vi "BackgroundCorrect.vi"(0 "Load Images":path=path "F:/pHGradienten/2015/150416_Bindungskurve_FeCN/500uW/15/a000000.tif", 1 "Load Background Images":path=path "F:/pHGradienten/2015/150218_ssDNA/ATTO488/50mer_2/a000000.tif", 2 "Image":dbl[][](graph), 3 "Frame":i32, 4 "Binning":dbl, 5 "Background Correction Mode:":T1(ring)=enum."Constant Value", 6 "# of Background image":i32=1499, 8 "Offset":dbl, 9 "Constant":dbl) -> (7 "Corrected Image":dbl[][](graph))   [LabVIEW 2010]
panel:
  out "Background Path in Folder":path[](array[path])=[path "F:/pHGradienten/2015/150416_Bindungskurve_FeCN/500uW/10/a000001.tif", path "F:/pHGradienten/2015/150416_Bindungskurve_FeCN/500uW/10/a000002.tif", path "F:/pHGradienten/2015/150416_Bindungskurve_FeCN/500uW/10/a000003.tif", path "F:/pHGradienten/2015/150416_Bindungskurve_FeCN/500uW/10/a000004.tif", path "F:/pHGradienten/2015/150416_Bindungskurve_FeCN/500uW/10/a000005.tif", path "F:/pHGradienten/2015/150416_Bindungskurve_FeCN/500uW/10/a000006.tif", path "F:/pHGradienten/2015/150416_Bindungskurve_FeCN/500uW/10/a000007.tif", path "F:/pHGradienten/2015/150416_Bindungskurve_FeCN/500uW/10/a000008.tif", path "F:/pHGradienten/2015/150416_Bindungskurve_FeCN/500uW/10/a000009.tif", path "F:/pHGradienten/2015/150416_Bindungskurve_FeCN/500uW/10/a000010.tif", path "F:/pHGradienten/2015/150416_Bindungskurve_FeCN/500uW/10/a000011.tif", path "F:/pHGradienten/2015/150416_Bindungskurve_FeCN/500uW/10/a000012.tif", path "F:/pHGradienten/2015/150416_Bindungskurve_FeCN/500uW/10/a000013.tif", path "F:/pHGradienten/2015/150416_Bindungskurve_FeCN/500uW/10/a000014.tif", path "F:/pHGradienten/2015/150416_Bindungskurve_FeCN/500uW/10/a000015.tif", path "F:/pHGradienten/2015/150416_Bindungskurve_FeCN/500uW/10/a000016.tif", path "F:/pHGradienten/2015/150416_Bindungskurve_FeCN/500uW/10/a000017.tif", path "F:/pHGradienten/2015/150416_Bindungskurve_FeCN/500uW/10/a000018.tif", path "F:/pHGradienten/2015/150416_Bindungskurve_FeCN/500uW/10/a000019.tif", path "F:/pHGradienten/2015/150416_Bindungskurve_FeCN/500uW/10/a000020.tif", path "F:/pHGradienten/2015/150416_Bindungskurve_FeCN/500uW/10/a000021.tif", path "F:/pHGradienten/2015/150416_Bindungskurve_FeCN/500uW/10/a000022.tif", path "F:/pHGradienten/2015/150416_Bindungskurve_FeCN/500uW/10/a000023.tif", path "F:/pHGradienten/2015/150416_Bindungskurve_FeCN/500uW/10/a000024.tif", path "F:/pHGradienten/2015/150416_Bindungskurve_FeCN/500uW/10/a000025.tif", path "F:/pHGradienten/2015/150416_Bindungskurve_FeCN/500uW/10/a000026.tif", path "F:/pHGradienten/2015/150416_Bindungskurve_FeCN/500uW/10/a000027.tif", path "F:/pHGradienten/2015/150416_Bindungskurve_FeCN/500uW/10/a000028.tif", path "F:/pHGradienten/2015/150416_Bindungskurve_FeCN/500uW/10/a000029.tif", path "F:/pHGradienten/2015/150416_Bindungskurve_FeCN/500uW/10/a000030.tif", path "F:/pHGradienten/2015/150416_Bindungskurve_FeCN/500uW/10/a000031.tif", path "F:/pHGradienten/2015/150416_Bindungskurve_FeCN/500uW/10/a000032.tif", path "F:/pHGradienten/2015/150416_Bindungskurve_FeCN/500uW/10/a000033.tif", path "F:/pHGradienten/2015/150416_Bindungskurve_FeCN/500uW/10/a000034.tif", path "F:/pHGradienten/2015/150416_Bindungskurve_FeCN/500uW/10/a000035.tif", path "F:/pHGradienten/2015/150416_Bindungskurve_FeCN/500uW/10/a000036.tif", path "F:/pHGradienten/2015/150416_Bindungskurve_FeCN/500uW/10/a000037.tif", path "F:/pHGradienten/2015/150416_Bindungskurve_FeCN/500uW/10/a000038.tif", path "F:/pHGradienten/2015/150416_Bindungskurve_FeCN/500uW/10/a000039.tif", path "F:/pHGradienten/2015/150416_Bindungskurve_FeCN/500uW/10/a000040.tif", path "F:/pHGradienten/2015/150416_Bindungskurve_FeCN/500uW/10/a000041.tif", path "F:/pHGradienten/2015/150416_Bindungskurve_FeCN/500uW/10/a000042.tif", path "F:/pHGradienten/2015/150416_Bindungskurve_FeCN/500uW/10/a000043.tif", path "F:/pHGradienten/2015/150416_Bindungskurve_FeCN/500uW/10/a000044.tif", path "F:/pHGradienten/2015/150416_Bindungskurve_FeCN/500uW/10/a000045.tif", path "F:/pHGradienten/2015/150416_Bindungskurve_FeCN/500uW/10/a000046.tif", path "F:/pHGradienten/2015/150416_Bindungskurve_FeCN/500uW/10/a000047.tif", path "F:/pHGradienten/2015/150416_Bindungskurve_FeCN/500uW/10/a000048.tif", path "F:/pHGradienten/2015/150416_Bindungskurve_FeCN/500uW/10/a000049.tif", path "F:/pHGradienten/2015/150416_Bindungskurve_FeCN/500uW/10/a000050.tif", path "F:/pHGradienten/2015/150416_Bindungskurve_FeCN/500uW/10/a000051.tif", path "F:/pHGradienten/2015/150416_Bindungskurve_FeCN/500uW/10/a000052.tif", path "F:/pHGradienten/2015/150416_Bindungskurve_FeCN/500uW/10/a000053.tif", path "F:/pHGradienten/2015/150416_Bindungskurve_FeCN/500uW/10/a000054.tif", path "F:/pHGradienten/2015/150416_Bindungskurve_FeCN/500uW/10/a000055.tif", path "F:/pHGradienten/2015/150416_Bindungskurve_FeCN/500uW/10/a000056.tif", path "F:/pHGradienten/2015/150416_Bindungskurve_FeCN/500uW/10/a000057.tif", path "F:/pHGradienten/2015/150416_Bindungskurve_FeCN/500uW/10/a000058.tif", path "F:/pHGradienten/2015/150416_Bindungskurve_FeCN/500uW/10/a000059.tif", path "F:/pHGradienten/2015/150416_Bindungskurve_FeCN/500uW/10/a000060.tif", path "F:/pHGradienten/2015/150416_Bindungskurve_FeCN/500uW/10/a000061.tif", path "F:/pHGradienten/2015/150416_Bindungskurve_FeCN/500uW/10/a000062.tif", path "F:/pHGradienten/2015/150416_Bindungskurve_FeCN/500uW/10/a000063.tif", path "F:/pHGradienten/2015/150416_Bindungskurve_FeCN/500uW/10/a000064.tif", path "F:/pHGradienten/2015/150416_Bindungskurve_FeCN/500uW/10/a000065.tif", path "F:/pHGradienten/2015/150416_Bindungskurve_FeCN/500uW/10/a000066.tif", path "F:/pHGradienten/2015/150416_Bindungskurve_FeCN/500uW/10/a000067.tif", path "F:/pHGradienten/2015/150416_Bindungskurve_FeCN/500uW/10/a000068.tif", path "F:/pHGradienten/2015/150416_Bindungskurve_FeCN/500uW/10/a000069.tif", path "F:/pHGradienten/2015/150416_Bindungskurve_FeCN/500uW/10/a000070.tif", path "F:/pHGradienten/2015/150416_Bindungskurve_FeCN/500uW/10/a000071.tif", path "F:/pHGradienten/2015/150416_Bindungskurve_FeCN/500uW/10/a000072.tif", path "F:/pHGradienten/2015/150416_Bindungskurve_FeCN/500uW/10/a000073.tif", path "F:/pHGradienten/2015/150416_Bindungskurve_FeCN/500uW/10/a000074.tif", path "F:/pHGradienten/2015/150416_Bindungskurve_FeCN/500uW/10/a000075.tif", path "F:/pHGradienten/2015/150416_Bindungskurve_FeCN/500uW/10/a000076.tif", path "F:/pHGradienten/2015/150416_Bindungskurve_FeCN/500uW/10/a000077.tif", path "F:/pHGradienten/2015/150416_Bindungskurve_FeCN/500uW/10/a000078.tif", path "F:/pHGradienten/2015/150416_Bindungskurve_FeCN/500uW/10/a000079.tif", path "F:/pHGradienten/2015/150416_Bindungskurve_FeCN/500uW/10/a000080.tif", path "F:/pHGradienten/2015/150416_Bindungskurve_FeCN/500uW/10/a000081.tif", path "F:/pHGradienten/2015/150416_Bindungskurve_FeCN/500uW/10/a000082.tif", path "F:/pHGradienten/2015/150416_Bindungskurve_FeCN/500uW/10/a000083.tif", path "F:/pHGradienten/2015/150416_Bindungskurve_FeCN/500uW/10/a000084.tif", path "F:/pHGradienten/2015/150416_Bindungskurve_FeCN/500uW/10/a000085.tif", path "F:/pHGradienten/2015/150416_Bindungskurve_FeCN/500uW/10/a000086.tif", path "F:/pHGradienten/2015/150416_Bindungskurve_FeCN/500uW/10/a000087.tif", path "F:/pHGradienten/2015/150416_Bindungskurve_FeCN/500uW/10/a000088.tif", path "F:/pHGradienten/2015/150416_Bindungskurve_FeCN/500uW/10/a000089.tif", path "F:/pHGradienten/2015/150416_Bindungskurve_FeCN/500uW/10/a000090.tif", path "F:/pHGradienten/2015/150416_Bindungskurve_FeCN/500uW/10/a000091.tif", path "F:/pHGradienten/2015/150416_Bindungskurve_FeCN/500uW/10/a000092.tif", path "F:/pHGradienten/2015/150416_Bindungskurve_FeCN/500uW/10/a000093.tif", path "F:/pHGradienten/2015/150416_Bindungskurve_FeCN/500uW/10/a000094.tif", path "F:/pHGradienten/2015/150416_Bindungskurve_FeCN/500uW/10/a000095.tif", path "F:/pHGradienten/2015/150416_Bindungskurve_FeCN/500uW/10/a000096.tif", path "F:/pHGradienten/2015/150416_Bindungskurve_FeCN/500uW/10/a000097.tif", path "F:/pHGradienten/2015/150416_Bindungskurve_FeCN/500uW/10/a000098.tif", path "F:/pHGradienten/2015/150416_Bindungskurve_FeCN/500uW/10/a000099.tif", path "F:/pHGradienten/2015/150416_Bindungskurve_FeCN/500uW/10/a000100.tif", path "F:/pHGradienten/2015/150416_Bindungskurve_FeCN/500uW/10/a000101.tif", path "F:/pHGradienten/2015/150416_Bindungskurve_FeCN/500uW/10/a000102.tif", path "F:/pHGradienten/2015/150416_Bindungskurve_FeCN/500uW/10/a000103.tif", path "F:/pHGradienten/2015/150416_Bindungskurve_FeCN/500uW/10/a000104.tif", path "F:/pHGradienten/2015/150416_Bindungskurve_FeCN/500uW/10/a000105.tif", path "F:/pHGradienten/2015/150416_Bindungskurve_FeCN/500uW/10/a000106.tif", path "F:/pHGradienten/2015/150416_Bindungskurve_FeCN/500uW/10/a000107.tif", path "F:/pHGradienten/2015/150416_Bindungskurve_FeCN/500uW/10/a000108.tif", path "F:/pHGradienten/2015/150416_Bindungskurve_FeCN/500uW/10/a000109.tif", path "F:/pHGradienten/2015/150416_Bindungskurve_FeCN/500uW/10/a000110.tif", path "F:/pHGradienten/2015/150416_Bindungskurve_FeCN/500uW/10/a000111.tif", path "F:/pHGradienten/2015/150416_Bindungskurve_FeCN/500uW/10/a000112.tif", path "F:/pHGradienten/2015/150416_Bindungskurve_FeCN/500uW/10/a000113.tif", path "F:/pHGradienten/2015/150416_Bindungskurve_FeCN/500uW/10/a000114.tif", path "F:/pHGradienten/2015/150416_Bindungskurve_FeCN/500uW/10/a000115.tif", path "F:/pHGradienten/2015/150416_Bindungskurve_FeCN/500uW/10/a000116.tif", path "F:/pHGradienten/2015/150416_Bindungskurve_FeCN/500uW/10/a000117.tif", path "F:/pHGradienten/2015/150416_Bindungskurve_FeCN/500uW/10/a000118.tif", path "F:/pHGradienten/2015/150416_Bindungskurve_FeCN/500uW/10/a000119.tif", path "F:/pHGradienten/2015/150416_Bindungskurve_FeCN/500uW/10/a000120.tif", path "F:/pHGradienten/2015/150416_Bindungskurve_FeCN/500uW/10/a000121.tif", path "F:/pHGradienten/2015/150416_Bindungskurve_FeCN/500uW/10/a000122.tif", path "F:/pHGradienten/2015/150416_Bindungskurve_FeCN/500uW/10/a000123.tif", path "F:/pHGradienten/2015/150416_Bindungskurve_FeCN/500uW/10/a000124.tif", path "F:/pHGradienten/2015/150416_Bindungskurve_FeCN/500uW/10/a000125.tif", path "F:/pHGradienten/2015/150416_Bindungskurve_FeCN/500uW/10/a000126.tif", path "F:/pHGradienten/2015/150416_Bindungskurve_FeCN/500uW/10/a000127.tif", path "F:/pHGradienten/2015/150416_Bindungskurve_FeCN/500uW/10/a000128.tif", path "F:/pHGradienten/2015/150416_Bindungskurve_FeCN/500uW/10/a000129.tif", path "F:/pHGradienten/2015/150416_Bindungskurve_FeCN/500uW/10/a000130.tif", path "F:/pHGradienten/2015/150416_Bindungskurve_FeCN/500uW/10/a000131.tif", path "F:/pHGradienten/2015/150416_Bindungskurve_FeCN/500uW/10/a000132.tif", path "F:/pHGradienten/2015/150416_Bindungskurve_FeCN/500uW/10/a000133.tif", path "F:/pHGradienten/2015/150416_Bindungskurve_FeCN/500uW/10/a000134.tif", path "F:/pHGradienten/2015/150416_Bindungskurve_FeCN/500uW/10/a000135.tif", path "F:/pHGradienten/2015/150416_Bindungskurve_FeCN/500uW/10/a000136.tif", path "F:/pHGradienten/2015/150416_Bindungskurve_FeCN/500uW/10/a000137.tif", path "F:/pHGradienten/2015/150416_Bindungskurve_FeCN/500uW/10/a000138.tif", path "F:/pHGradienten/2015/150416_Bindungskurve_FeCN/500uW/10/a000139.tif", path "F:/pHGradienten/2015/150416_Bindungskurve_FeCN/500uW/10/a000140.tif", path "F:/pHGradienten/2015/150416_Bindungskurve_FeCN/500uW/10/a000141.tif", path "F:/pHGradienten/2015/150416_Bindungskurve_FeCN/500uW/10/a000142.tif", path "F:/pHGradienten/2015/150416_Bindungskurve_FeCN/500uW/10/a000143.tif", path "F:/pHGradienten/2015/150416_Bindungskurve_FeCN/500uW/10/a000144.tif", path "F:/pHGradienten/2015/150416_Bindungskurve_FeCN/500uW/10/a000145.tif", path "F:/pHGradienten/2015/150416_Bindungskurve_FeCN/500uW/10/a000146.tif", path "F:/pHGradienten/2015/150416_Bindungskurve_FeCN/500uW/10/a000147.tif", path "F:/pHGradienten/2015/150416_Bindungskurve_FeCN/500uW/10/a000148.tif", path "F:/pHGradienten/2015/150416_Bindungskurve_FeCN/500uW/10/a000149.tif", path "F:/pHGradienten/2015/150416_Bindungskurve_FeCN/500uW/10/a000150.tif", path "F:/pHGradienten/2015/150416_Bindungskurve_FeCN/500uW/10/a000151.tif", path "F:/pHGradienten/2015/150416_Bindungskurve_FeCN/500uW/10/a000152.tif", path "F:/pHGradienten/2015/150416_Bindungskurve_FeCN/500uW/10/a000153.tif", path "F:/pHGradienten/2015/150416_Bindungskurve_FeCN/500uW/10/a000154.tif", path "F:/pHGradienten/2015/150416_Bindungskurve_FeCN/500uW/10/a000155.tif", path "F:/pHGradienten/2015/150416_Bindungskurve_FeCN/500uW/10/a000156.tif", path "F:/pHGradienten/2015/150416_Bindungskurve_FeCN/500uW/10/a000157.tif", path "F:/pHGradienten/2015/150416_Bindungskurve_FeCN/500uW/10/a000158.tif", path "F:/pHGradienten/2015/150416_Bindungskurve_FeCN/500uW/10/a000159.tif", path "F:/pHGradienten/2015/150416_Bindungskurve_FeCN/500uW/10/a000160.tif", path "F:/pHGradienten/2015/150416_Bindungskurve_FeCN/500uW/10/a000161.tif", path "F:/pHGradienten/2015/150416_Bindungskurve_FeCN/500uW/10/a000162.tif", path "F:/pHGradienten/2015/150416_Bindungskurve_FeCN/500uW/10/a000163.tif", path "F:/pHGradienten/2015/150416_Bindungskurve_FeCN/500uW/10/a000164.tif", path "F:/pHGradienten/2015/150416_Bindungskurve_FeCN/500uW/10/a000165.tif", path "F:/pHGradienten/2015/150416_Bindungskurve_FeCN/500uW/10/a000166.tif", path "F:/pHGradienten/2015/150416_Bindungskurve_FeCN/500uW/10/a000167.tif", path "F:/pHGradienten/2015/150416_Bindungskurve_FeCN/500uW/10/a000168.tif", path "F:/pHGradienten/2015/150416_Bindungskurve_FeCN/500uW/10/a000169.tif", path "F:/pHGradienten/2015/150416_Bindungskurve_FeCN/500uW/10/a000170.tif", path "F:/pHGradienten/2015/150416_Bindungskurve_FeCN/500uW/10/a000171.tif", path "F:/pHGradienten/2015/150416_Bindungskurve_FeCN/500uW/10/a000172.tif", path "F:/pHGradienten/2015/150416_Bindungskurve_FeCN/500uW/10/a000173.tif", path "F:/pHGradienten/2015/150416_Bindungskurve_FeCN/500uW/10/a000174.tif", path "F:/pHGradienten/2015/150416_Bindungskurve_FeCN/500uW/10/a000175.tif", path "F:/pHGradienten/2015/150416_Bindungskurve_FeCN/500uW/10/a000176.tif", path "F:/pHGradienten/2015/150416_Bindungskurve_FeCN/500uW/10/a000177.tif", path "F:/pHGradienten/2015/150416_Bindungskurve_FeCN/500uW/10/a000178.tif", path "F:/pHGradienten/2015/150416_Bindungskurve_FeCN/500uW/10/a000179.tif", path "F:/pHGradienten/2015/150416_Bindungskurve_FeCN/500uW/10/a000180.tif", path "F:/pHGradienten/2015/150416_Bindungskurve_FeCN/500uW/10/a000181.tif", path "F:/pHGradienten/2015/150416_Bindungskurve_FeCN/500uW/10/a000182.tif", path "F:/pHGradienten/2015/150416_Bindungskurve_FeCN/500uW/10/a000183.tif", path "F:/pHGradienten/2015/150416_Bindungskurve_FeCN/500uW/10/a000184.tif", path "F:/pHGradienten/2015/150416_Bindungskurve_FeCN/500uW/10/a000185.tif", path "F:/pHGradienten/2015/150416_Bindungskurve_FeCN/500uW/10/a000186.tif", path "F:/pHGradienten/2015/150416_Bindungskurve_FeCN/500uW/10/a000187.tif", path "F:/pHGradienten/2015/150416_Bindungskurve_FeCN/500uW/10/a000188.tif", path "F:/pHGradienten/2015/150416_Bindungskurve_FeCN/500uW/10/a000189.tif", path "F:/pHGradienten/2015/150416_Bindungskurve_FeCN/500uW/10/a000190.tif", path "F:/pHGradienten/2015/150416_Bindungskurve_FeCN/500uW/10/a000191.tif", path "F:/pHGradienten/2015/150416_Bindungskurve_FeCN/500uW/10/a000192.tif", path "F:/pHGradienten/2015/150416_Bindungskurve_FeCN/500uW/10/a000193.tif", path "F:/pHGradienten/2015/150416_Bindungskurve_FeCN/500uW/10/a000194.tif", path "F:/pHGradienten/2015/150416_Bindungskurve_FeCN/500uW/10/a000195.tif", path "F:/pHGradienten/2015/150416_Bindungskurve_FeCN/500uW/10/a000196.tif", path "F:/pHGradienten/2015/150416_Bindungskurve_FeCN/500uW/10/a000197.tif", path "F:/pHGradienten/2015/150416_Bindungskurve_FeCN/500uW/10/a000198.tif", path "F:/pHGradienten/2015/150416_Bindungskurve_FeCN/500uW/10/a000199.tif", path "F:/pHGradienten/2015/150416_Bindungskurve_FeCN/500uW/10/a000200.tif", path "F:/pHGradienten/2015/150416_Bindungskurve_FeCN/500uW/10/a000201.tif", path "F:/pHGradienten/2015/150416_Bindungskurve_FeCN/500uW/10/a000202.tif", path "F:/pHGradienten/2015/150416_Bindungskurve_FeCN/500uW/10/a000203.tif", path "F:/pHGradienten/2015/150416_Bindungskurve_FeCN/500uW/10/a000204.tif", path "F:/pHGradienten/2015/150416_Bindungskurve_FeCN/500uW/10/a000205.tif", path "F:/pHGradienten/2015/150416_Bindungskurve_FeCN/500uW/10/a000206.tif", path "F:/pHGradienten/2015/150416_Bindungskurve_FeCN/500uW/10/a000207.tif", path "F:/pHGradienten/2015/150416_Bindungskurve_FeCN/500uW/10/a000208.tif", path "F:/pHGradienten/2015/150416_Bindungskurve_FeCN/500uW/10/a000209.tif", path "F:/pHGradienten/2015/150416_Bindungskurve_FeCN/500uW/10/a000210.tif", path "F:/pHGradienten/2015/150416_Bindungskurve_FeCN/500uW/10/a000211.tif", path "F:/pHGradienten/2015/150416_Bindungskurve_FeCN/500uW/10/a000212.tif", path "F:/pHGradienten/2015/150416_Bindungskurve_FeCN/500uW/10/a000213.tif", path "F:/pHGradienten/2015/150416_Bindungskurve_FeCN/500uW/10/a000214.tif", path "F:/pHGradienten/2015/150416_Bindungskurve_FeCN/500uW/10/a000215.tif", path "F:/pHGradienten/2015/150416_Bindungskurve_FeCN/500uW/10/a000216.tif", path "F:/pHGradienten/2015/150416_Bindungskurve_FeCN/500uW/10/a000217.tif", path "F:/pHGradienten/2015/150416_Bindungskurve_FeCN/500uW/10/a000218.tif", path "F:/pHGradienten/2015/150416_Bindungskurve_FeCN/500uW/10/a000219.tif", path "F:/pHGradienten/2015/150416_Bindungskurve_FeCN/500uW/10/a000220.tif", path "F:/pHGradienten/2015/150416_Bindungskurve_FeCN/500uW/10/a000221.tif", path "F:/pHGradienten/2015/150416_Bindungskurve_FeCN/500uW/10/a000222.tif", path "F:/pHGradienten/2015/150416_Bindungskurve_FeCN/500uW/10/a000223.tif", path "F:/pHGradienten/2015/150416_Bindungskurve_FeCN/500uW/10/a000224.tif", path "F:/pHGradienten/2015/150416_Bindungskurve_FeCN/500uW/10/a000225.tif", path "F:/pHGradienten/2015/150416_Bindungskurve_FeCN/500uW/10/a000226.tif", path "F:/pHGradienten/2015/150416_Bindungskurve_FeCN/500uW/10/a000227.tif", path "F:/pHGradienten/2015/150416_Bindungskurve_FeCN/500uW/10/a000228.tif", path "F:/pHGradienten/2015/150416_Bindungskurve_FeCN/500uW/10/a000229.tif", path "F:/pHGradienten/2015/150416_Bindungskurve_FeCN/500uW/10/a000230.tif", path "F:/pHGradienten/2015/150416_Bindungskurve_FeCN/500uW/10/a000231.tif", path "F:/pHGradienten/2015/150416_Bindungskurve_FeCN/500uW/10/a000232.tif", path "F:/pHGradienten/2015/150416_Bindungskurve_FeCN/500uW/10/a000233.tif", path "F:/pHGradienten/2015/150416_Bindungskurve_FeCN/500uW/10/a000234.tif", path "F:/pHGradienten/2015/150416_Bindungskurve_FeCN/500uW/10/a000235.tif", path "F:/pHGradienten/2015/150416_Bindungskurve_FeCN/500uW/10/a000236.tif", path "F:/pHGradienten/2015/150416_Bindungskurve_FeCN/500uW/10/a000237.tif", path "F:/pHGradienten/2015/150416_Bindungskurve_FeCN/500uW/10/a000238.tif", path "F:/pHGradienten/2015/150416_Bindungskurve_FeCN/500uW/10/a000239.tif", path "F:/pHGradienten/2015/150416_Bindungskurve_FeCN/500uW/10/a000240.tif", path "F:/pHGradienten/2015/150416_Bindungskurve_FeCN/500uW/10/a000241.tif", path "F:/pHGradienten/2015/150416_Bindungskurve_FeCN/500uW/10/a000242.tif", path "F:/pHGradienten/2015/150416_Bindungskurve_FeCN/500uW/10/a000243.tif", path "F:/pHGradienten/2015/150416_Bindungskurve_FeCN/500uW/10/a000244.tif", path "F:/pHGradienten/2015/150416_Bindungskurve_FeCN/500uW/10/a000245.tif", path "F:/pHGradienten/2015/150416_Bindungskurve_FeCN/500uW/10/a000246.tif", path "F:/pHGradienten/2015/150416_Bindungskurve_FeCN/500uW/10/a000247.tif", path "F:/pHGradienten/2015/150416_Bindungskurve_FeCN/500uW/10/a000248.tif", path "F:/pHGradienten/2015/150416_Bindungskurve_FeCN/500uW/10/a000249.tif", path "F:/pHGradienten/2015/150416_Bindungskurve_FeCN/500uW/10/a000250.tif", path "F:/pHGradienten/2015/150416_Bindungskurve_FeCN/500uW/10/a000251.tif", path "F:/pHGradienten/2015/150416_Bindungskurve_FeCN/500uW/10/a000252.tif", path "F:/pHGradienten/2015/150416_Bindungskurve_FeCN/500uW/10/a000253.tif", path "F:/pHGradienten/2015/150416_Bindungskurve_FeCN/500uW/10/a000254.tif", path "F:/pHGradienten/2015/150416_Bindungskurve_FeCN/500uW/10/a000255.tif", path "F:/pHGradienten/2015/150416_Bindungskurve_FeCN/500uW/10/a000256.tif", path "F:/pHGradienten/2015/150416_Bindungskurve_FeCN/500uW/10/a000257.tif", path "F:/pHGradienten/2015/150416_Bindungskurve_FeCN/500uW/10/a000258.tif", path "F:/pHGradienten/2015/150416_Bindungskurve_FeCN/500uW/10/a000259.tif", path "F:/pHGradienten/2015/150416_Bindungskurve_FeCN/500uW/10/a000260.tif", path "F:/pHGradienten/2015/150416_Bindungskurve_FeCN/500uW/10/a000261.tif", path "F:/pHGradienten/2015/150416_Bindungskurve_FeCN/500uW/10/a000262.tif", path "F:/pHGradienten/2015/150416_Bindungskurve_FeCN/500uW/10/a000263.tif", path "F:/pHGradienten/2015/150416_Bindungskurve_FeCN/500uW/10/a000264.tif", path "F:/pHGradienten/2015/150416_Bindungskurve_FeCN/500uW/10/a000265.tif", path "F:/pHGradienten/2015/150416_Bindungskurve_FeCN/500uW/10/a000266.tif", path "F:/pHGradienten/2015/150416_Bindungskurve_FeCN/500uW/10/a000267.tif", path "F:/pHGradienten/2015/150416_Bindungskurve_FeCN/500uW/10/a000268.tif", path "F:/pHGradienten/2015/150416_Bindungskurve_FeCN/500uW/10/a000269.tif", path "F:/pHGradienten/2015/150416_Bindungskurve_FeCN/500uW/10/a000270.tif", path "F:/pHGradienten/2015/150416_Bindungskurve_FeCN/500uW/10/a000271.tif", path "F:/pHGradienten/2015/150416_Bindungskurve_FeCN/500uW/10/a000272.tif", path "F:/pHGradienten/2015/150416_Bindungskurve_FeCN/500uW/10/a000273.tif", path "F:/pHGradienten/2015/150416_Bindungskurve_FeCN/500uW/10/a000274.tif", path "F:/pHGradienten/2015/150416_Bindungskurve_FeCN/500uW/10/a000275.tif", path "F:/pHGradienten/2015/150416_Bindungskurve_FeCN/500uW/10/a000276.tif", path "F:/pHGradienten/2015/150416_Bindungskurve_FeCN/500uW/10/a000277.tif", path "F:/pHGradienten/2015/150416_Bindungskurve_FeCN/500uW/10/a000278.tif", path "F:/pHGradienten/2015/150416_Bindungskurve_FeCN/500uW/10/a000279.tif", path "F:/pHGradienten/2015/150416_Bindungskurve_FeCN/500uW/10/a000280.tif", path "F:/pHGradienten/2015/150416_Bindungskurve_FeCN/500uW/10/a000281.tif", path "F:/pHGradienten/2015/150416_Bindungskurve_FeCN/500uW/10/a000282.tif", path "F:/pHGradienten/2015/150416_Bindungskurve_FeCN/500uW/10/a000283.tif", path "F:/pHGradienten/2015/150416_Bindungskurve_FeCN/500uW/10/a000284.tif", path "F:/pHGradienten/2015/150416_Bindungskurve_FeCN/500uW/10/a000285.tif", path "F:/pHGradienten/2015/150416_Bindungskurve_FeCN/500uW/10/a000286.tif", path "F:/pHGradienten/2015/150416_Bindungskurve_FeCN/500uW/10/a000287.tif", path "F:/pHGradienten/2015/150416_Bindungskurve_FeCN/500uW/10/a000288.tif", path "F:/pHGradienten/2015/150416_Bindungskurve_FeCN/500uW/10/a000289.tif", path "F:/pHGradienten/2015/150416_Bindungskurve_FeCN/500uW/10/a000290.tif", path "F:/pHGradienten/2015/150416_Bindungskurve_FeCN/500uW/10/a000291.tif", path "F:/pHGradienten/2015/150416_Bindungskurve_FeCN/500uW/10/a000292.tif", path "F:/pHGradienten/2015/150416_Bindungskurve_FeCN/500uW/10/a000293.tif", path "F:/pHGradienten/2015/150416_Bindungskurve_FeCN/500uW/10/a000294.tif", path "F:/pHGradienten/2015/150416_Bindungskurve_FeCN/500uW/10/a000295.tif", path "F:/pHGradienten/2015/150416_Bindungskurve_FeCN/500uW/10/a000296.tif", path "F:/pHGradienten/2015/150416_Bindungskurve_FeCN/500uW/10/a000297.tif", path "F:/pHGradienten/2015/150416_Bindungskurve_FeCN/500uW/10/a000298.tif", path "F:/pHGradienten/2015/150416_Bindungskurve_FeCN/500uW/10/a000299.tif", path "F:/pHGradienten/2015/150416_Bindungskurve_FeCN/500uW/10/a000300.tif", path "F:/pHGradienten/2015/150416_Bindungskurve_FeCN/500uW/10/a000301.tif", path "F:/pHGradienten/2015/150416_Bindungskurve_FeCN/500uW/10/a000302.tif", path "F:/pHGradienten/2015/150416_Bindungskurve_FeCN/500uW/10/a000303.tif", path "F:/pHGradienten/2015/150416_Bindungskurve_FeCN/500uW/10/a000304.tif", path "F:/pHGradienten/2015/150416_Bindungskurve_FeCN/500uW/10/a000305.tif", path "F:/pHGradienten/2015/150416_Bindungskurve_FeCN/500uW/10/a000306.tif", path "F:/pHGradienten/2015/150416_Bindungskurve_FeCN/500uW/10/a000307.tif", path "F:/pHGradienten/2015/150416_Bindungskurve_FeCN/500uW/10/a000308.tif", path "F:/pHGradienten/2015/150416_Bindungskurve_FeCN/500uW/10/a000309.tif", path "F:/pHGradienten/2015/150416_Bindungskurve_FeCN/500uW/10/a000310.tif", path "F:/pHGradienten/2015/150416_Bindungskurve_FeCN/500uW/10/a000311.tif", path "F:/pHGradienten/2015/150416_Bindungskurve_FeCN/500uW/10/a000312.tif", path "F:/pHGradienten/2015/150416_Bindungskurve_FeCN/500uW/10/a000313.tif", path "F:/pHGradienten/2015/150416_Bindungskurve_FeCN/500uW/10/a000314.tif", path "F:/pHGradienten/2015/150416_Bindungskurve_FeCN/500uW/10/a000315.tif", path "F:/pHGradienten/2015/150416_Bindungskurve_FeCN/500uW/10/a000316.tif", path "F:/pHGradienten/2015/150416_Bindungskurve_FeCN/500uW/10/a000317.tif", path "F:/pHGradienten/2015/150416_Bindungskurve_FeCN/500uW/10/a000318.tif", path "F:/pHGradienten/2015/150416_Bindungskurve_FeCN/500uW/10/a000319.tif", path "F:/pHGradienten/2015/150416_Bindungskurve_FeCN/500uW/10/a000320.tif", path "F:/pHGradienten/2015/150416_Bindungskurve_FeCN/500uW/10/a000321.tif", path "F:/pHGradienten/2015/150416_Bindungskurve_FeCN/500uW/10/a000322.tif", path "F:/pHGradienten/2015/150416_Bindungskurve_FeCN/500uW/10/a000323.tif", path "F:/pHGradienten/2015/150416_Bindungskurve_FeCN/500uW/10/a000324.tif", path "F:/pHGradienten/2015/150416_Bindungskurve_FeCN/500uW/10/a000325.tif", path "F:/pHGradienten/2015/150416_Bindungskurve_FeCN/500uW/10/a000326.tif", path "F:/pHGradienten/2015/150416_Bindungskurve_FeCN/500uW/10/a000327.tif", path "F:/pHGradienten/2015/150416_Bindungskurve_FeCN/500uW/10/a000328.tif", path "F:/pHGradienten/2015/150416_Bindungskurve_FeCN/500uW/10/a000329.tif", path "F:/pHGradienten/2015/150416_Bindungskurve_FeCN/500uW/10/a000330.tif", path "F:/pHGradienten/2015/150416_Bindungskurve_FeCN/500uW/10/a000331.tif", path "F:/pHGradienten/2015/150416_Bindungskurve_FeCN/500uW/10/a000332.tif", path "F:/pHGradienten/2015/150416_Bindungskurve_FeCN/500uW/10/a000333.tif", path "F:/pHGradienten/2015/150416_Bindungskurve_FeCN/500uW/10/a000334.tif", path "F:/pHGradienten/2015/150416_Bindungskurve_FeCN/500uW/10/a000335.tif", path "F:/pHGradienten/2015/150416_Bindungskurve_FeCN/500uW/10/a000336.tif", path "F:/pHGradienten/2015/150416_Bindungskurve_FeCN/500uW/10/a000337.tif", path "F:/pHGradienten/2015/150416_Bindungskurve_FeCN/500uW/10/a000338.tif", path "F:/pHGradienten/2015/150416_Bindungskurve_FeCN/500uW/10/a000339.tif", path "F:/pHGradienten/2015/150416_Bindungskurve_FeCN/500uW/10/a000340.tif", path "F:/pHGradienten/2015/150416_Bindungskurve_FeCN/500uW/10/a000341.tif", path "F:/pHGradienten/2015/150416_Bindungskurve_FeCN/500uW/10/a000342.tif", path "F:/pHGradienten/2015/150416_Bindungskurve_FeCN/500uW/10/a000343.tif", path "F:/pHGradienten/2015/150416_Bindungskurve_FeCN/500uW/10/a000344.tif", path "F:/pHGradienten/2015/150416_Bindungskurve_FeCN/500uW/10/a000345.tif", path "F:/pHGradienten/2015/150416_Bindungskurve_FeCN/500uW/10/a000346.tif", path "F:/pHGradienten/2015/150416_Bindungskurve_FeCN/500uW/10/a000347.tif", path "F:/pHGradienten/2015/150416_Bindungskurve_FeCN/500uW/10/a000348.tif", path "F:/pHGradienten/2015/150416_Bindungskurve_FeCN/500uW/10/a000349.tif", path "F:/pHGradienten/2015/150416_Bindungskurve_FeCN/500uW/10/a000350.tif", path "F:/pHGradienten/2015/150416_Bindungskurve_FeCN/500uW/10/a000351.tif", path "F:/pHGradienten/2015/150416_Bindungskurve_FeCN/500uW/10/a000352.tif", path "F:/pHGradienten/2015/150416_Bindungskurve_FeCN/500uW/10/a000353.tif", path "F:/pHGradienten/2015/150416_Bindungskurve_FeCN/500uW/10/a000354.tif", path "F:/pHGradienten/2015/150416_Bindungskurve_FeCN/500uW/10/a000355.tif", path "F:/pHGradienten/2015/150416_Bindungskurve_FeCN/500uW/10/a000356.tif", path "F:/pHGradienten/2015/150416_Bindungskurve_FeCN/500uW/10/a000357.tif", path "F:/pHGradienten/2015/150416_Bindungskurve_FeCN/500uW/10/a000358.tif", path "F:/pHGradienten/2015/150416_Bindungskurve_FeCN/500uW/10/a000359.tif", path "F:/pHGradienten/2015/150416_Bindungskurve_FeCN/500uW/10/a000360.tif", path "F:/pHGradienten/2015/150416_Bindungskurve_FeCN/500uW/10/a000361.tif", path "F:/pHGradienten/2015/150416_Bindungskurve_FeCN/500uW/10/a000362.tif", path "F:/pHGradienten/2015/150416_Bindungskurve_FeCN/500uW/10/a000363.tif", path "F:/pHGradienten/2015/150416_Bindungskurve_FeCN/500uW/10/a000364.tif", path "F:/pHGradienten/2015/150416_Bindungskurve_FeCN/500uW/10/a000365.tif", path "F:/pHGradienten/2015/150416_Bindungskurve_FeCN/500uW/10/a000366.tif", path "F:/pHGradienten/2015/150416_Bindungskurve_FeCN/500uW/10/a000367.tif", path "F:/pHGradienten/2015/150416_Bindungskurve_FeCN/500uW/10/a000368.tif", path "F:/pHGradienten/2015/150416_Bindungskurve_FeCN/500uW/10/a000369.tif", path "F:/pHGradienten/2015/150416_Bindungskurve_FeCN/500uW/10/a000370.tif", path "F:/pHGradienten/2015/150416_Bindungskurve_FeCN/500uW/10/a000371.tif", path "F:/pHGradienten/2015/150416_Bindungskurve_FeCN/500uW/10/a000372.tif", path "F:/pHGradienten/2015/150416_Bindungskurve_FeCN/500uW/10/a000373.tif", path "F:/pHGradienten/2015/150416_Bindungskurve_FeCN/500uW/10/a000374.tif", path "F:/pHGradienten/2015/150416_Bindungskurve_FeCN/500uW/10/a000375.tif", path "F:/pHGradienten/2015/150416_Bindungskurve_FeCN/500uW/10/a000376.tif", path "F:/pHGradienten/2015/150416_Bindungskurve_FeCN/500uW/10/a000377.tif", path "F:/pHGradienten/2015/150416_Bindungskurve_FeCN/500uW/10/a000378.tif", path "F:/pHGradienten/2015/150416_Bindungskurve_FeCN/500uW/10/a000379.tif", path "F:/pHGradienten/2015/150416_Bindungskurve_FeCN/500uW/10/a000380.tif", path "F:/pHGradienten/2015/150416_Bindungskurve_FeCN/500uW/10/a000381.tif", path "F:/pHGradienten/2015/150416_Bindungskurve_FeCN/500uW/10/a000382.tif", path "F:/pHGradienten/2015/150416_Bindungskurve_FeCN/500uW/10/a000383.tif", path "F:/pHGradienten/2015/150416_Bindungskurve_FeCN/500uW/10/a000384.tif", path "F:/pHGradienten/2015/150416_Bindungskurve_FeCN/500uW/10/a000385.tif", path "F:/pHGradienten/2015/150416_Bindungskurve_FeCN/500uW/10/a000386.tif", path "F:/pHGradienten/2015/150416_Bindungskurve_FeCN/500uW/10/a000387.tif", path "F:/pHGradienten/2015/150416_Bindungskurve_FeCN/500uW/10/a000388.tif", path "F:/pHGradienten/2015/150416_Bindungskurve_FeCN/500uW/10/a000389.tif", path "F:/pHGradienten/2015/150416_Bindungskurve_FeCN/500uW/10/a000390.tif", path "F:/pHGradienten/2015/150416_Bindungskurve_FeCN/500uW/10/a000391.tif", path "F:/pHGradienten/2015/150416_Bindungskurve_FeCN/500uW/10/a000392.tif", path "F:/pHGradienten/2015/150416_Bindungskurve_FeCN/500uW/10/a000393.tif", path "F:/pHGradienten/2015/150416_Bindungskurve_FeCN/500uW/10/a000394.tif", path "F:/pHGradienten/2015/150416_Bindungskurve_FeCN/500uW/10/a000395.tif", path "F:/pHGradienten/2015/150416_Bindungskurve_FeCN/500uW/10/a000396.tif", path "F:/pHGradienten/2015/150416_Bindungskurve_FeCN/500uW/10/a000397.tif", path "F:/pHGradienten/2015/150416_Bindungskurve_FeCN/500uW/10/a000398.tif", path "F:/pHGradienten/2015/150416_Bindungskurve_FeCN/500uW/10/a000399.tif", path "F:/pHGradienten/2015/150416_Bindungskurve_FeCN/500uW/10/a000400.tif", path "F:/pHGradienten/2015/150416_Bindungskurve_FeCN/500uW/10/a000401.tif", path "F:/pHGradienten/2015/150416_Bindungskurve_FeCN/500uW/10/a000402.tif", path "F:/pHGradienten/2015/150416_Bindungskurve_FeCN/500uW/10/a000403.tif", path "F:/pHGradienten/2015/150416_Bindungskurve_FeCN/500uW/10/a000404.tif", path "F:/pHGradienten/2015/150416_Bindungskurve_FeCN/500uW/10/a000405.tif", path "F:/pHGradienten/2015/150416_Bindungskurve_FeCN/500uW/10/a000406.tif", path "F:/pHGradienten/2015/150416_Bindungskurve_FeCN/500uW/10/a000407.tif", path "F:/pHGradienten/2015/150416_Bindungskurve_FeCN/500uW/10/a000408.tif", path "F:/pHGradienten/2015/150416_Bindungskurve_FeCN/500uW/10/a000409.tif", path "F:/pHGradienten/2015/150416_Bindungskurve_FeCN/500uW/10/a000410.tif", path "F:/pHGradienten/2015/150416_Bindungskurve_FeCN/500uW/10/a000411.tif", path "F:/pHGradienten/2015/150416_Bindungskurve_FeCN/500uW/10/a000412.tif", path "F:/pHGradienten/2015/150416_Bindungskurve_FeCN/500uW/10/a000413.tif", path "F:/pHGradienten/2015/150416_Bindungskurve_FeCN/500uW/10/a000414.tif", path "F:/pHGradienten/2015/150416_Bindungskurve_FeCN/500uW/10/a000415.tif", path "F:/pHGradienten/2015/150416_Bindungskurve_FeCN/500uW/10/a000416.tif", path "F:/pHGradienten/2015/150416_Bindungskurve_FeCN/500uW/10/a000417.tif", path "F:/pHGradienten/2015/150416_Bindungskurve_FeCN/500uW/10/a000418.tif", path "F:/pHGradienten/2015/150416_Bindungskurve_FeCN/500uW/10/a000419.tif", path "F:/pHGradienten/2015/150416_Bindungskurve_FeCN/500uW/10/a000420.tif", path "F:/pHGradienten/2015/150416_Bindungskurve_FeCN/500uW/10/a000421.tif", path "F:/pHGradienten/2015/150416_Bindungskurve_FeCN/500uW/10/a000422.tif", path "F:/pHGradienten/2015/150416_Bindungskurve_FeCN/500uW/10/a000423.tif", path "F:/pHGradienten/2015/150416_Bindungskurve_FeCN/500uW/10/a000424.tif", path "F:/pHGradienten/2015/150416_Bindungskurve_FeCN/500uW/10/a000425.tif", path "F:/pHGradienten/2015/150416_Bindungskurve_FeCN/500uW/10/a000426.tif", path "F:/pHGradienten/2015/150416_Bindungskurve_FeCN/500uW/10/a000427.tif", path "F:/pHGradienten/2015/150416_Bindungskurve_FeCN/500uW/10/a000428.tif", path "F:/pHGradienten/2015/150416_Bindungskurve_FeCN/500uW/10/a000429.tif", path "F:/pHGradienten/2015/150416_Bindungskurve_FeCN/500uW/10/a000430.tif", path "F:/pHGradienten/2015/150416_Bindungskurve_FeCN/500uW/10/a000431.tif", path "F:/pHGradienten/2015/150416_Bindungskurve_FeCN/500uW/10/a000432.tif", path "F:/pHGradienten/2015/150416_Bindungskurve_FeCN/500uW/10/a000433.tif", path "F:/pHGradienten/2015/150416_Bindungskurve_FeCN/500uW/10/a000434.tif", path "F:/pHGradienten/2015/150416_Bindungskurve_FeCN/500uW/10/a000435.tif", path "F:/pHGradienten/2015/150416_Bindungskurve_FeCN/500uW/10/a000436.tif", path "F:/pHGradienten/2015/150416_Bindungskurve_FeCN/500uW/10/a000437.tif", path "F:/pHGradienten/2015/150416_Bindungskurve_FeCN/500uW/10/a000438.tif", path "F:/pHGradienten/2015/150416_Bindungskurve_FeCN/500uW/10/a000439.tif", path "F:/pHGradienten/2015/150416_Bindungskurve_FeCN/500uW/10/a000440.tif", path "F:/pHGradienten/2015/150416_Bindungskurve_FeCN/500uW/10/a000441.tif", path "F:/pHGradienten/2015/150416_Bindungskurve_FeCN/500uW/10/a000442.tif", path "F:/pHGradienten/2015/150416_Bindungskurve_FeCN/500uW/10/a000443.tif", path "F:/pHGradienten/2015/150416_Bindungskurve_FeCN/500uW/10/a000444.tif", path "F:/pHGradienten/2015/150416_Bindungskurve_FeCN/500uW/10/a000445.tif", path "F:/pHGradienten/2015/150416_Bindungskurve_FeCN/500uW/10/a000446.tif", path "F:/pHGradienten/2015/150416_Bindungskurve_FeCN/500uW/10/a000447.tif", path "F:/pHGradienten/2015/150416_Bindungskurve_FeCN/500uW/10/a000448.tif", path "F:/pHGradienten/2015/150416_Bindungskurve_FeCN/500uW/10/a000449.tif", path "F:/pHGradienten/2015/150416_Bindungskurve_FeCN/500uW/10/a000450.tif", path "F:/pHGradienten/2015/150416_Bindungskurve_FeCN/500uW/10/a000451.tif", path "F:/pHGradienten/2015/150416_Bindungskurve_FeCN/500uW/10/a000452.tif", path "F:/pHGradienten/2015/150416_Bindungskurve_FeCN/500uW/10/a000453.tif", path "F:/pHGradienten/2015/150416_Bindungskurve_FeCN/500uW/10/a000454.tif", path "F:/pHGradienten/2015/150416_Bindungskurve_FeCN/500uW/10/a000455.tif", path "F:/pHGradienten/2015/150416_Bindungskurve_FeCN/500uW/10/a000456.tif", path "F:/pHGradienten/2015/150416_Bindungskurve_FeCN/500uW/10/a000457.tif", path "F:/pHGradienten/2015/150416_Bindungskurve_FeCN/500uW/10/a000458.tif", path "F:/pHGradienten/2015/150416_Bindungskurve_FeCN/500uW/10/a000459.tif", path "F:/pHGradienten/2015/150416_Bindungskurve_FeCN/500uW/10/a000460.tif", path "F:/pHGradienten/2015/150416_Bindungskurve_FeCN/500uW/10/a000461.tif", path "F:/pHGradienten/2015/150416_Bindungskurve_FeCN/500uW/10/a000462.tif", path "F:/pHGradienten/2015/150416_Bindungskurve_FeCN/500uW/10/a000463.tif", path "F:/pHGradienten/2015/150416_Bindungskurve_FeCN/500uW/10/a000464.tif", path "F:/pHGradienten/2015/150416_Bindungskurve_FeCN/500uW/10/a000465.tif", path "F:/pHGradienten/2015/150416_Bindungskurve_FeCN/500uW/10/a000466.tif", path "F:/pHGradienten/2015/150416_Bindungskurve_FeCN/500uW/10/a000467.tif", path "F:/pHGradienten/2015/150416_Bindungskurve_FeCN/500uW/10/a000468.tif", path "F:/pHGradienten/2015/150416_Bindungskurve_FeCN/500uW/10/a000469.tif", path "F:/pHGradienten/2015/150416_Bindungskurve_FeCN/500uW/10/a000470.tif", path "F:/pHGradienten/2015/150416_Bindungskurve_FeCN/500uW/10/a000471.tif", path "F:/pHGradienten/2015/150416_Bindungskurve_FeCN/500uW/10/a000472.tif", path "F:/pHGradienten/2015/150416_Bindungskurve_FeCN/500uW/10/a000473.tif", path "F:/pHGradienten/2015/150416_Bindungskurve_FeCN/500uW/10/a000474.tif", path "F:/pHGradienten/2015/150416_Bindungskurve_FeCN/500uW/10/a000475.tif", path "F:/pHGradienten/2015/150416_Bindungskurve_FeCN/500uW/10/a000476.tif", path "F:/pHGradienten/2015/150416_Bindungskurve_FeCN/500uW/10/a000477.tif", path "F:/pHGradienten/2015/150416_Bindungskurve_FeCN/500uW/10/a000478.tif", path "F:/pHGradienten/2015/150416_Bindungskurve_FeCN/500uW/10/a000479.tif", path "F:/pHGradienten/2015/150416_Bindungskurve_FeCN/500uW/10/a000480.tif", path "F:/pHGradienten/2015/150416_Bindungskurve_FeCN/500uW/10/a000481.tif", path "F:/pHGradienten/2015/150416_Bindungskurve_FeCN/500uW/10/a000482.tif", path "F:/pHGradienten/2015/150416_Bindungskurve_FeCN/500uW/10/a000483.tif", path "F:/pHGradienten/2015/150416_Bindungskurve_FeCN/500uW/10/a000484.tif", path "F:/pHGradienten/2015/150416_Bindungskurve_FeCN/500uW/10/a000485.tif", path "F:/pHGradienten/2015/150416_Bindungskurve_FeCN/500uW/10/a000486.tif", path "F:/pHGradienten/2015/150416_Bindungskurve_FeCN/500uW/10/a000487.tif", path "F:/pHGradienten/2015/150416_Bindungskurve_FeCN/500uW/10/a000488.tif", path "F:/pHGradienten/2015/150416_Bindungskurve_FeCN/500uW/10/a000489.tif", path "F:/pHGradienten/2015/150416_Bindungskurve_FeCN/500uW/10/a000490.tif", path "F:/pHGradienten/2015/150416_Bindungskurve_FeCN/500uW/10/a000491.tif", path "F:/pHGradienten/2015/150416_Bindungskurve_FeCN/500uW/10/a000492.tif", path "F:/pHGradienten/2015/150416_Bindungskurve_FeCN/500uW/10/a000493.tif", path "F:/pHGradienten/2015/150416_Bindungskurve_FeCN/500uW/10/a000494.tif", path "F:/pHGradienten/2015/150416_Bindungskurve_FeCN/500uW/10/a000495.tif", path "F:/pHGradienten/2015/150416_Bindungskurve_FeCN/500uW/10/a000496.tif", path "F:/pHGradienten/2015/150416_Bindungskurve_FeCN/500uW/10/a000497.tif", path "F:/pHGradienten/2015/150416_Bindungskurve_FeCN/500uW/10/a000498.tif", path "F:/pHGradienten/2015/150416_Bindungskurve_FeCN/500uW/10/a000499.tif", path "F:/pHGradienten/2015/150416_Bindungskurve_FeCN/500uW/10/a000500.tif", path "F:/pHGradienten/2015/150416_Bindungskurve_FeCN/500uW/10/a000501.tif", path "F:/pHGradienten/2015/150416_Bindungskurve_FeCN/500uW/10/a000502.tif", path "F:/pHGradienten/2015/150416_Bindungskurve_FeCN/500uW/10/a000503.tif", path "F:/pHGradienten/2015/150416_Bindungskurve_FeCN/500uW/10/a000504.tif", path "F:/pHGradienten/2015/150416_Bindungskurve_FeCN/500uW/10/a000505.tif", path "F:/pHGradienten/2015/150416_Bindungskurve_FeCN/500uW/10/a000506.tif", path "F:/pHGradienten/2015/150416_Bindungskurve_FeCN/500uW/10/a000507.tif", path "F:/pHGradienten/2015/150416_Bindungskurve_FeCN/500uW/10/a000508.tif", path "F:/pHGradienten/2015/150416_Bindungskurve_FeCN/500uW/10/a000509.tif", path "F:/pHGradienten/2015/150416_Bindungskurve_FeCN/500uW/10/a000510.tif", path "F:/pHGradienten/2015/150416_Bindungskurve_FeCN/500uW/10/a000511.tif", path "F:/pHGradienten/2015/150416_Bindungskurve_FeCN/500uW/10/a000512.tif", path "F:/pHGradienten/2015/150416_Bindungskurve_FeCN/500uW/10/a000513.tif", path "F:/pHGradienten/2015/150416_Bindungskurve_FeCN/500uW/10/a000514.tif", path "F:/pHGradienten/2015/150416_Bindungskurve_FeCN/500uW/10/a000515.tif", path "F:/pHGradienten/2015/150416_Bindungskurve_FeCN/500uW/10/a000516.tif", path "F:/pHGradienten/2015/150416_Bindungskurve_FeCN/500uW/10/a000517.tif", path "F:/pHGradienten/2015/150416_Bindungskurve_FeCN/500uW/10/a000518.tif", path "F:/pHGradienten/2015/150416_Bindungskurve_FeCN/500uW/10/a000519.tif", path "F:/pHGradienten/2015/150416_Bindungskurve_FeCN/500uW/10/a000520.tif", path "F:/pHGradienten/2015/150416_Bindungskurve_FeCN/500uW/10/a000521.tif", path "F:/pHGradienten/2015/150416_Bindungskurve_FeCN/500uW/10/a000522.tif", path "F:/pHGradienten/2015/150416_Bindungskurve_FeCN/500uW/10/a000523.tif", path "F:/pHGradienten/2015/150416_Bindungskurve_FeCN/500uW/10/a000524.tif", path "F:/pHGradienten/2015/150416_Bindungskurve_FeCN/500uW/10/a000525.tif", path "F:/pHGradienten/2015/150416_Bindungskurve_FeCN/500uW/10/a000526.tif", path "F:/pHGradienten/2015/150416_Bindungskurve_FeCN/500uW/10/a000527.tif", path "F:/pHGradienten/2015/150416_Bindungskurve_FeCN/500uW/10/a000528.tif", path "F:/pHGradienten/2015/150416_Bindungskurve_FeCN/500uW/10/a000529.tif", path "F:/pHGradienten/2015/150416_Bindungskurve_FeCN/500uW/10/a000530.tif", path "F:/pHGradienten/2015/150416_Bindungskurve_FeCN/500uW/10/a000531.tif", path "F:/pHGradienten/2015/150416_Bindungskurve_FeCN/500uW/10/a000532.tif", path "F:/pHGradienten/2015/150416_Bindungskurve_FeCN/500uW/10/a000533.tif", path "F:/pHGradienten/2015/150416_Bindungskurve_FeCN/500uW/10/a000534.tif", path "F:/pHGradienten/2015/150416_Bindungskurve_FeCN/500uW/10/a000535.tif", path "F:/pHGradienten/2015/150416_Bindungskurve_FeCN/500uW/10/a000536.tif", path "F:/pHGradienten/2015/150416_Bindungskurve_FeCN/500uW/10/a000537.tif", path "F:/pHGradienten/2015/150416_Bindungskurve_FeCN/500uW/10/a000538.tif", path "F:/pHGradienten/2015/150416_Bindungskurve_FeCN/500uW/10/a000539.tif", path "F:/pHGradienten/2015/150416_Bindungskurve_FeCN/500uW/10/a000540.tif", path "F:/pHGradienten/2015/150416_Bindungskurve_FeCN/500uW/10/a000541.tif", path "F:/pHGradienten/2015/150416_Bindungskurve_FeCN/500uW/10/a000542.tif", path "F:/pHGradienten/2015/150416_Bindungskurve_FeCN/500uW/10/a000543.tif", path "F:/pHGradienten/2015/150416_Bindungskurve_FeCN/500uW/10/a000544.tif", path "F:/pHGradienten/2015/150416_Bindungskurve_FeCN/500uW/10/a000545.tif", path "F:/pHGradienten/2015/150416_Bindungskurve_FeCN/500uW/10/a000546.tif", path "F:/pHGradienten/2015/150416_Bindungskurve_FeCN/500uW/10/a000547.tif", path "F:/pHGradienten/2015/150416_Bindungskurve_FeCN/500uW/10/a000548.tif", path "F:/pHGradienten/2015/150416_Bindungskurve_FeCN/500uW/10/a000549.tif", path "F:/pHGradienten/2015/150416_Bindungskurve_FeCN/500uW/10/a000550.tif", path "F:/pHGradienten/2015/150416_Bindungskurve_FeCN/500uW/10/a000551.tif", path "F:/pHGradienten/2015/150416_Bindungskurve_FeCN/500uW/10/a000552.tif", path "F:/pHGradienten/2015/150416_Bindungskurve_FeCN/500uW/10/a000553.tif", path "F:/pHGradienten/2015/150416_Bindungskurve_FeCN/500uW/10/a000554.tif", path "F:/pHGradienten/2015/150416_Bindungskurve_FeCN/500uW/10/a000555.tif", path "F:/pHGradienten/2015/150416_Bindungskurve_FeCN/500uW/10/a000556.tif", path "F:/pHGradienten/2015/150416_Bindungskurve_FeCN/500uW/10/a000557.tif", path "F:/pHGradienten/2015/150416_Bindungskurve_FeCN/500uW/10/a000558.tif", path "F:/pHGradienten/2015/150416_Bindungskurve_FeCN/500uW/10/a000559.tif", path "F:/pHGradienten/2015/150416_Bindungskurve_FeCN/500uW/10/a000560.tif", path "F:/pHGradienten/2015/150416_Bindungskurve_FeCN/500uW/10/a000561.tif", path "F:/pHGradienten/2015/150416_Bindungskurve_FeCN/500uW/10/a000562.tif", path "F:/pHGradienten/2015/150416_Bindungskurve_FeCN/500uW/10/a000563.tif", path "F:/pHGradienten/2015/150416_Bindungskurve_FeCN/500uW/10/a000564.tif", path "F:/pHGradienten/2015/150416_Bindungskurve_FeCN/500uW/10/a000565.tif", path "F:/pHGradienten/2015/150416_Bindungskurve_FeCN/500uW/10/a000566.tif", path "F:/pHGradienten/2015/150416_Bindungskurve_FeCN/500uW/10/a000567.tif", path "F:/pHGradienten/2015/150416_Bindungskurve_FeCN/500uW/10/a000568.tif", path "F:/pHGradienten/2015/150416_Bindungskurve_FeCN/500uW/10/a000569.tif", path "F:/pHGradienten/2015/150416_Bindungskurve_FeCN/500uW/10/a000570.tif", path "F:/pHGradienten/2015/150416_Bindungskurve_FeCN/500uW/10/a000571.tif", path "F:/pHGradienten/2015/150416_Bindungskurve_FeCN/500uW/10/a000572.tif", path "F:/pHGradienten/2015/150416_Bindungskurve_FeCN/500uW/10/a000573.tif", path "F:/pHGradienten/2015/150416_Bindungskurve_FeCN/500uW/10/a000574.tif", path "F:/pHGradienten/2015/150416_Bindungskurve_FeCN/500uW/10/a000575.tif", path "F:/pHGradienten/2015/150416_Bindungskurve_FeCN/500uW/10/a000576.tif", path "F:/pHGradienten/2015/150416_Bindungskurve_FeCN/500uW/10/a000577.tif", path "F:/pHGradienten/2015/150416_Bindungskurve_FeCN/500uW/10/a000578.tif", path "F:/pHGradienten/2015/150416_Bindungskurve_FeCN/500uW/10/a000579.tif", path "F:/pHGradienten/2015/150416_Bindungskurve_FeCN/500uW/10/a000580.tif", path "F:/pHGradienten/2015/150416_Bindungskurve_FeCN/500uW/10/a000581.tif", path "F:/pHGradienten/2015/150416_Bindungskurve_FeCN/500uW/10/a000582.tif", path "F:/pHGradienten/2015/150416_Bindungskurve_FeCN/500uW/10/a000583.tif", path "F:/pHGradienten/2015/150416_Bindungskurve_FeCN/500uW/10/a000584.tif", path "F:/pHGradienten/2015/150416_Bindungskurve_FeCN/500uW/10/a000585.tif", path "F:/pHGradienten/2015/150416_Bindungskurve_FeCN/500uW/10/a000586.tif", path "F:/pHGradienten/2015/150416_Bindungskurve_FeCN/500uW/10/a000587.tif", path "F:/pHGradienten/2015/150416_Bindungskurve_FeCN/500uW/10/a000588.tif", path "F:/pHGradienten/2015/150416_Bindungskurve_FeCN/500uW/10/a000589.tif", path "F:/pHGradienten/2015/150416_Bindungskurve_FeCN/500uW/10/a000590.tif", path "F:/pHGradienten/2015/150416_Bindungskurve_FeCN/500uW/10/a000591.tif", path "F:/pHGradienten/2015/150416_Bindungskurve_FeCN/500uW/10/a000592.tif", path "F:/pHGradienten/2015/150416_Bindungskurve_FeCN/500uW/10/a000593.tif", path "F:/pHGradienten/2015/150416_Bindungskurve_FeCN/500uW/10/a000594.tif", path "F:/pHGradienten/2015/150416_Bindungskurve_FeCN/500uW/10/a000595.tif", path "F:/pHGradienten/2015/150416_Bindungskurve_FeCN/500uW/10/a000596.tif", path "F:/pHGradienten/2015/150416_Bindungskurve_FeCN/500uW/10/a000597.tif", path "F:/pHGradienten/2015/150416_Bindungskurve_FeCN/500uW/10/a000598.tif", path "F:/pHGradienten/2015/150416_Bindungskurve_FeCN/500uW/10/a000599.tif", path "F:/pHGradienten/2015/150416_Bindungskurve_FeCN/500uW/10/a000600.tif", path "F:/pHGradienten/2015/150416_Bindungskurve_FeCN/500uW/10/a000601.tif", path "F:/pHGradienten/2015/150416_Bindungskurve_FeCN/500uW/10/a000602.tif", path "F:/pHGradienten/2015/150416_Bindungskurve_FeCN/500uW/10/a000603.tif", path "F:/pHGradienten/2015/150416_Bindungskurve_FeCN/500uW/10/a000604.tif", path "F:/pHGradienten/2015/150416_Bindungskurve_FeCN/500uW/10/a000605.tif", path "F:/pHGradienten/2015/150416_Bindungskurve_FeCN/500uW/10/a000606.tif", path "F:/pHGradienten/2015/150416_Bindungskurve_FeCN/500uW/10/a000607.tif", path "F:/pHGradienten/2015/150416_Bindungskurve_FeCN/500uW/10/a000608.tif", path "F:/pHGradienten/2015/150416_Bindungskurve_FeCN/500uW/10/a000609.tif", path "F:/pHGradienten/2015/150416_Bindungskurve_FeCN/500uW/10/a000610.tif", path "F:/pHGradienten/2015/150416_Bindungskurve_FeCN/500uW/10/a000611.tif", path "F:/pHGradienten/2015/150416_Bindungskurve_FeCN/500uW/10/a000612.tif", path "F:/pHGradienten/2015/150416_Bindungskurve_FeCN/500uW/10/a000613.tif", path "F:/pHGradienten/2015/150416_Bindungskurve_FeCN/500uW/10/a000614.tif", path "F:/pHGradienten/2015/150416_Bindungskurve_FeCN/500uW/10/a000615.tif", path "F:/pHGradienten/2015/150416_Bindungskurve_FeCN/500uW/10/a000616.tif", path "F:/pHGradienten/2015/150416_Bindungskurve_FeCN/500uW/10/a000617.tif", path "F:/pHGradienten/2015/150416_Bindungskurve_FeCN/500uW/10/a000618.tif", path "F:/pHGradienten/2015/150416_Bindungskurve_FeCN/500uW/10/a000619.tif", path "F:/pHGradienten/2015/150416_Bindungskurve_FeCN/500uW/10/a000620.tif", path "F:/pHGradienten/2015/150416_Bindungskurve_FeCN/500uW/10/a000621.tif", path "F:/pHGradienten/2015/150416_Bindungskurve_FeCN/500uW/10/a000622.tif", path "F:/pHGradienten/2015/150416_Bindungskurve_FeCN/500uW/10/a000623.tif", path "F:/pHGradienten/2015/150416_Bindungskurve_FeCN/500uW/10/a000624.tif", path "F:/pHGradienten/2015/150416_Bindungskurve_FeCN/500uW/10/a000625.tif", path "F:/pHGradienten/2015/150416_Bindungskurve_FeCN/500uW/10/a000626.tif", path "F:/pHGradienten/2015/150416_Bindungskurve_FeCN/500uW/10/a000627.tif", path "F:/pHGradienten/2015/150416_Bindungskurve_FeCN/500uW/10/a000628.tif", path "F:/pHGradienten/2015/150416_Bindungskurve_FeCN/500uW/10/a000629.tif", path "F:/pHGradienten/2015/150416_Bindungskurve_FeCN/500uW/10/a000630.tif", path "F:/pHGradienten/2015/150416_Bindungskurve_FeCN/500uW/10/a000631.tif", path "F:/pHGradienten/2015/150416_Bindungskurve_FeCN/500uW/10/a000632.tif", path "F:/pHGradienten/2015/150416_Bindungskurve_FeCN/500uW/10/a000633.tif", path "F:/pHGradienten/2015/150416_Bindungskurve_FeCN/500uW/10/a000634.tif", path "F:/pHGradienten/2015/150416_Bindungskurve_FeCN/500uW/10/a000635.tif", path "F:/pHGradienten/2015/150416_Bindungskurve_FeCN/500uW/10/a000636.tif", path "F:/pHGradienten/2015/150416_Bindungskurve_FeCN/500uW/10/a000637.tif", path "F:/pHGradienten/2015/150416_Bindungskurve_FeCN/500uW/10/a000638.tif", path "F:/pHGradienten/2015/150416_Bindungskurve_FeCN/500uW/10/a000639.tif", path "F:/pHGradienten/2015/150416_Bindungskurve_FeCN/500uW/10/a000640.tif", path "F:/pHGradienten/2015/150416_Bindungskurve_FeCN/500uW/10/a000641.tif", path "F:/pHGradienten/2015/150416_Bindungskurve_FeCN/500uW/10/a000642.tif", path "F:/pHGradienten/2015/150416_Bindungskurve_FeCN/500uW/10/a000643.tif", path "F:/pHGradienten/2015/150416_Bindungskurve_FeCN/500uW/10/a000644.tif", path "F:/pHGradienten/2015/150416_Bindungskurve_FeCN/500uW/10/a000645.tif", path "F:/pHGradienten/2015/150416_Bindungskurve_FeCN/500uW/10/a000646.tif", path "F:/pHGradienten/2015/150416_Bindungskurve_FeCN/500uW/10/a000647.tif", path "F:/pHGradienten/2015/150416_Bindungskurve_FeCN/500uW/10/a000648.tif", path "F:/pHGradienten/2015/150416_Bindungskurve_FeCN/500uW/10/a000649.tif", path "F:/pHGradienten/2015/150416_Bindungskurve_FeCN/500uW/10/a000650.tif", path "F:/pHGradienten/2015/150416_Bindungskurve_FeCN/500uW/10/a000651.tif", path "F:/pHGradienten/2015/150416_Bindungskurve_FeCN/500uW/10/a000652.tif", path "F:/pHGradienten/2015/150416_Bindungskurve_FeCN/500uW/10/a000653.tif", path "F:/pHGradienten/2015/150416_Bindungskurve_FeCN/500uW/10/a000654.tif", path "F:/pHGradienten/2015/150416_Bindungskurve_FeCN/500uW/10/a000655.tif", path "F:/pHGradienten/2015/150416_Bindungskurve_FeCN/500uW/10/a000656.tif", path "F:/pHGradienten/2015/150416_Bindungskurve_FeCN/500uW/10/a000657.tif", path "F:/pHGradienten/2015/150416_Bindungskurve_FeCN/500uW/10/a000658.tif", path "F:/pHGradienten/2015/150416_Bindungskurve_FeCN/500uW/10/a000659.tif", path "F:/pHGradienten/2015/150416_Bindungskurve_FeCN/500uW/10/a000660.tif", path "F:/pHGradienten/2015/150416_Bindungskurve_FeCN/500uW/10/a000661.tif", path "F:/pHGradienten/2015/150416_Bindungskurve_FeCN/500uW/10/a000662.tif", path "F:/pHGradienten/2015/150416_Bindungskurve_FeCN/500uW/10/a000663.tif", path "F:/pHGradienten/2015/150416_Bindungskurve_FeCN/500uW/10/a000664.tif", path "F:/pHGradienten/2015/150416_Bindungskurve_FeCN/500uW/10/a000665.tif", path "F:/pHGradienten/2015/150416_Bindungskurve_FeCN/500uW/10/a000666.tif", path "F:/pHGradienten/2015/150416_Bindungskurve_FeCN/500uW/10/a000667.tif", path "F:/pHGradienten/2015/150416_Bindungskurve_FeCN/500uW/10/a000668.tif", path "F:/pHGradienten/2015/150416_Bindungskurve_FeCN/500uW/10/a000669.tif", path "F:/pHGradienten/2015/150416_Bindungskurve_FeCN/500uW/10/a000670.tif", path "F:/pHGradienten/2015/150416_Bindungskurve_FeCN/500uW/10/a000671.tif", path "F:/pHGradienten/2015/150416_Bindungskurve_FeCN/500uW/10/a000672.tif", path "F:/pHGradienten/2015/150416_Bindungskurve_FeCN/500uW/10/a000673.tif", path "F:/pHGradienten/2015/150416_Bindungskurve_FeCN/500uW/10/a000674.tif", path "F:/pHGradienten/2015/150416_Bindungskurve_FeCN/500uW/10/a000675.tif", path "F:/pHGradienten/2015/150416_Bindungskurve_FeCN/500uW/10/a000676.tif", path "F:/pHGradienten/2015/150416_Bindungskurve_FeCN/500uW/10/a000677.tif", path "F:/pHGradienten/2015/150416_Bindungskurve_FeCN/500uW/10/a000678.tif", path "F:/pHGradienten/2015/150416_Bindungskurve_FeCN/500uW/10/a000679.tif", path "F:/pHGradienten/2015/150416_Bindungskurve_FeCN/500uW/10/a000680.tif", path "F:/pHGradienten/2015/150416_Bindungskurve_FeCN/500uW/10/a000681.tif", path "F:/pHGradienten/2015/150416_Bindungskurve_FeCN/500uW/10/a000682.tif", path "F:/pHGradienten/2015/150416_Bindungskurve_FeCN/500uW/10/a000683.tif", path "F:/pHGradienten/2015/150416_Bindungskurve_FeCN/500uW/10/a000684.tif", path "F:/pHGradienten/2015/150416_Bindungskurve_FeCN/500uW/10/a000685.tif", path "F:/pHGradienten/2015/150416_Bindungskurve_FeCN/500uW/10/a000686.tif", path "F:/pHGradienten/2015/150416_Bindungskurve_FeCN/500uW/10/a000687.tif", path "F:/pHGradienten/2015/150416_Bindungskurve_FeCN/500uW/10/a000688.tif", path "F:/pHGradienten/2015/150416_Bindungskurve_FeCN/500uW/10/a000689.tif", path "F:/pHGradienten/2015/150416_Bindungskurve_FeCN/500uW/10/a000690.tif", path "F:/pHGradienten/2015/150416_Bindungskurve_FeCN/500uW/10/a000691.tif", path "F:/pHGradienten/2015/150416_Bindungskurve_FeCN/500uW/10/a000692.tif", path "F:/pHGradienten/2015/150416_Bindungskurve_FeCN/500uW/10/a000693.tif", path "F:/pHGradienten/2015/150416_Bindungskurve_FeCN/500uW/10/a000694.tif", path "F:/pHGradienten/2015/150416_Bindungskurve_FeCN/500uW/10/a000695.tif", path "F:/pHGradienten/2015/150416_Bindungskurve_FeCN/500uW/10/a000696.tif", path "F:/pHGradienten/2015/150416_Bindungskurve_FeCN/500uW/10/a000697.tif", path "F:/pHGradienten/2015/150416_Bindungskurve_FeCN/500uW/10/a000698.tif", path "F:/pHGradienten/2015/150416_Bindungskurve_FeCN/500uW/10/a000699.tif", path "F:/pHGradienten/2015/150416_Bindungskurve_FeCN/500uW/10/a000700.tif", path "F:/pHGradienten/2015/150416_Bindungskurve_FeCN/500uW/10/a000701.tif", path "F:/pHGradienten/2015/150416_Bindungskurve_FeCN/500uW/10/a000702.tif", path "F:/pHGradienten/2015/150416_Bindungskurve_FeCN/500uW/10/a000703.tif", path "F:/pHGradienten/2015/150416_Bindungskurve_FeCN/500uW/10/a000704.tif", path "F:/pHGradienten/2015/150416_Bindungskurve_FeCN/500uW/10/a000705.tif", path "F:/pHGradienten/2015/150416_Bindungskurve_FeCN/500uW/10/a000706.tif", path "F:/pHGradienten/2015/150416_Bindungskurve_FeCN/500uW/10/a000707.tif", path "F:/pHGradienten/2015/150416_Bindungskurve_FeCN/500uW/10/a000708.tif", path "F:/pHGradienten/2015/150416_Bindungskurve_FeCN/500uW/10/a000709.tif", path "F:/pHGradienten/2015/150416_Bindungskurve_FeCN/500uW/10/a000710.tif", path "F:/pHGradienten/2015/150416_Bindungskurve_FeCN/500uW/10/a000711.tif", path "F:/pHGradienten/2015/150416_Bindungskurve_FeCN/500uW/10/a000712.tif", path "F:/pHGradienten/2015/150416_Bindungskurve_FeCN/500uW/10/a000713.tif", path "F:/pHGradienten/2015/150416_Bindungskurve_FeCN/500uW/10/a000714.tif", path "F:/pHGradienten/2015/150416_Bindungskurve_FeCN/500uW/10/a000715.tif", path "F:/pHGradienten/2015/150416_Bindungskurve_FeCN/500uW/10/a000716.tif", path "F:/pHGradienten/2015/150416_Bindungskurve_FeCN/500uW/10/a000717.tif", path "F:/pHGradienten/2015/150416_Bindungskurve_FeCN/500uW/10/a000718.tif", path "F:/pHGradienten/2015/150416_Bindungskurve_FeCN/500uW/10/a000719.tif", path "F:/pHGradienten/2015/150416_Bindungskurve_FeCN/500uW/10/a000720.tif", path "F:/pHGradienten/2015/150416_Bindungskurve_FeCN/500uW/10/a000721.tif", path "F:/pHGradienten/2015/150416_Bindungskurve_FeCN/500uW/10/a000722.tif", path "F:/pHGradienten/2015/150416_Bindungskurve_FeCN/500uW/10/a000723.tif", path "F:/pHGradienten/2015/150416_Bindungskurve_FeCN/500uW/10/a000724.tif", path "F:/pHGradienten/2015/150416_Bindungskurve_FeCN/500uW/10/a000725.tif", path "F:/pHGradienten/2015/150416_Bindungskurve_FeCN/500uW/10/a000726.tif", path "F:/pHGradienten/2015/150416_Bindungskurve_FeCN/500uW/10/a000727.tif", path "F:/pHGradienten/2015/150416_Bindungskurve_FeCN/500uW/10/a000728.tif", path "F:/pHGradienten/2015/150416_Bindungskurve_FeCN/500uW/10/a000729.tif", path "F:/pHGradienten/2015/150416_Bindungskurve_FeCN/500uW/10/a000730.tif", path "F:/pHGradienten/2015/150416_Bindungskurve_FeCN/500uW/10/a000731.tif", path "F:/pHGradienten/2015/150416_Bindungskurve_FeCN/500uW/10/a000732.tif", path "F:/pHGradienten/2015/150416_Bindungskurve_FeCN/500uW/10/a000733.tif", path "F:/pHGradienten/2015/150416_Bindungskurve_FeCN/500uW/10/a000734.tif", path "F:/pHGradienten/2015/150416_Bindungskurve_FeCN/500uW/10/a000735.tif", path "F:/pHGradienten/2015/150416_Bindungskurve_FeCN/500uW/10/a000736.tif", path "F:/pHGradienten/2015/150416_Bindungskurve_FeCN/500uW/10/a000737.tif", path "F:/pHGradienten/2015/150416_Bindungskurve_FeCN/500uW/10/a000738.tif", path "F:/pHGradienten/2015/150416_Bindungskurve_FeCN/500uW/10/a000739.tif", path "F:/pHGradienten/2015/150416_Bindungskurve_FeCN/500uW/10/a000740.tif", path "F:/pHGradienten/2015/150416_Bindungskurve_FeCN/500uW/10/a000741.tif", path "F:/pHGradienten/2015/150416_Bindungskurve_FeCN/500uW/10/a000742.tif", path "F:/pHGradienten/2015/150416_Bindungskurve_FeCN/500uW/10/a000743.tif", path "F:/pHGradienten/2015/150416_Bindungskurve_FeCN/500uW/10/a000744.tif", path "F:/pHGradienten/2015/150416_Bindungskurve_FeCN/500uW/10/a000745.tif", path "F:/pHGradienten/2015/150416_Bindungskurve_FeCN/500uW/10/a000746.tif", path "F:/pHGradienten/2015/150416_Bindungskurve_FeCN/500uW/10/a000747.tif", path "F:/pHGradienten/2015/150416_Bindungskurve_FeCN/500uW/10/a000748.tif", path "F:/pHGradienten/2015/150416_Bindungskurve_FeCN/500uW/10/a000749.tif", path "F:/pHGradienten/2015/150416_Bindungskurve_FeCN/500uW/10/a000750.tif", path "F:/pHGradienten/2015/150416_Bindungskurve_FeCN/500uW/10/a000751.tif", path "F:/pHGradienten/2015/150416_Bindungskurve_FeCN/500uW/10/a000752.tif", path "F:/pHGradienten/2015/150416_Bindungskurve_FeCN/500uW/10/a000753.tif", path "F:/pHGradienten/2015/150416_Bindungskurve_FeCN/500uW/10/a000754.tif", path "F:/pHGradienten/2015/150416_Bindungskurve_FeCN/500uW/10/a000755.tif", path "F:/pHGradienten/2015/150416_Bindungskurve_FeCN/500uW/10/a000756.tif", path "F:/pHGradienten/2015/150416_Bindungskurve_FeCN/500uW/10/a000757.tif", path "F:/pHGradienten/2015/150416_Bindungskurve_FeCN/500uW/10/a000758.tif", path "F:/pHGradienten/2015/150416_Bindungskurve_FeCN/500uW/10/a000759.tif", path "F:/pHGradienten/2015/150416_Bindungskurve_FeCN/500uW/10/a000760.tif", path "F:/pHGradienten/2015/150416_Bindungskurve_FeCN/500uW/10/a000761.tif", path "F:/pHGradienten/2015/150416_Bindungskurve_FeCN/500uW/10/a000762.tif", path "F:/pHGradienten/2015/150416_Bindungskurve_FeCN/500uW/10/a000763.tif", path "F:/pHGradienten/2015/150416_Bindungskurve_FeCN/500uW/10/a000764.tif", path "F:/pHGradienten/2015/150416_Bindungskurve_FeCN/500uW/10/a000765.tif", path "F:/pHGradienten/2015/150416_Bindungskurve_FeCN/500uW/10/a000766.tif", path "F:/pHGradienten/2015/150416_Bindungskurve_FeCN/500uW/10/a000767.tif", path "F:/pHGradienten/2015/150416_Bindungskurve_FeCN/500uW/10/a000768.tif", path "F:/pHGradienten/2015/150416_Bindungskurve_FeCN/500uW/10/a000769.tif", path "F:/pHGradienten/2015/150416_Bindungskurve_FeCN/500uW/10/a000770.tif", path "F:/pHGradienten/2015/150416_Bindungskurve_FeCN/500uW/10/a000771.tif", path "F:/pHGradienten/2015/150416_Bindungskurve_FeCN/500uW/10/a000772.tif", path "F:/pHGradienten/2015/150416_Bindungskurve_FeCN/500uW/10/a000773.tif", path "F:/pHGradienten/2015/150416_Bindungskurve_FeCN/500uW/10/a000774.tif", path "F:/pHGradienten/2015/150416_Bindungskurve_FeCN/500uW/10/a000775.tif", path "F:/pHGradienten/2015/150416_Bindungskurve_FeCN/500uW/10/a000776.tif", path "F:/pHGradienten/2015/150416_Bindungskurve_FeCN/500uW/10/a000777.tif", path "F:/pHGradienten/2015/150416_Bindungskurve_FeCN/500uW/10/a000778.tif", path "F:/pHGradienten/2015/150416_Bindungskurve_FeCN/500uW/10/a000779.tif", path "F:/pHGradienten/2015/150416_Bindungskurve_FeCN/500uW/10/a000780.tif", path "F:/pHGradienten/2015/150416_Bindungskurve_FeCN/500uW/10/a000781.tif", path "F:/pHGradienten/2015/150416_Bindungskurve_FeCN/500uW/10/a000782.tif", path "F:/pHGradienten/2015/150416_Bindungskurve_FeCN/500uW/10/a000783.tif", path "F:/pHGradienten/2015/150416_Bindungskurve_FeCN/500uW/10/a000784.tif", path "F:/pHGradienten/2015/150416_Bindungskurve_FeCN/500uW/10/a000785.tif", path "F:/pHGradienten/2015/150416_Bindungskurve_FeCN/500uW/10/a000786.tif", path "F:/pHGradienten/2015/150416_Bindungskurve_FeCN/500uW/10/a000787.tif", path "F:/pHGradienten/2015/150416_Bindungskurve_FeCN/500uW/10/a000788.tif", path "F:/pHGradienten/2015/150416_Bindungskurve_FeCN/500uW/10/a000789.tif", path "F:/pHGradienten/2015/150416_Bindungskurve_FeCN/500uW/10/a000790.tif", path "F:/pHGradienten/2015/150416_Bindungskurve_FeCN/500uW/10/a000791.tif", path "F:/pHGradienten/2015/150416_Bindungskurve_FeCN/500uW/10/a000792.tif", path "F:/pHGradienten/2015/150416_Bindungskurve_FeCN/500uW/10/a000793.tif", path "F:/pHGradienten/2015/150416_Bindungskurve_FeCN/500uW/10/a000794.tif", path "F:/pHGradienten/2015/150416_Bindungskurve_FeCN/500uW/10/a000795.tif", path "F:/pHGradienten/2015/150416_Bindungskurve_FeCN/500uW/10/a000796.tif", path "F:/pHGradienten/2015/150416_Bindungskurve_FeCN/500uW/10/a000797.tif", path "F:/pHGradienten/2015/150416_Bindungskurve_FeCN/500uW/10/a000798.tif", path "F:/pHGradienten/2015/150416_Bindungskurve_FeCN/500uW/10/a000799.tif", path "F:/pHGradienten/2015/150416_Bindungskurve_FeCN/500uW/10/a000800.tif", path "F:/pHGradienten/2015/150416_Bindungskurve_FeCN/500uW/10/a000801.tif", path "F:/pHGradienten/2015/150416_Bindungskurve_FeCN/500uW/10/a000802.tif", path "F:/pHGradienten/2015/150416_Bindungskurve_FeCN/500uW/10/a000803.tif", path "F:/pHGradienten/2015/150416_Bindungskurve_FeCN/500uW/10/a000804.tif", path "F:/pHGradienten/2015/150416_Bindungskurve_FeCN/500uW/10/a000805.tif", path "F:/pHGradienten/2015/150416_Bindungskurve_FeCN/500uW/10/a000806.tif", path "F:/pHGradienten/2015/150416_Bindungskurve_FeCN/500uW/10/a000807.tif", path "F:/pHGradienten/2015/150416_Bindungskurve_FeCN/500uW/10/a000808.tif", path "F:/pHGradienten/2015/150416_Bindungskurve_FeCN/500uW/10/a000809.tif", path "F:/pHGradienten/2015/150416_Bindungskurve_FeCN/500uW/10/a000810.tif", path "F:/pHGradienten/2015/150416_Bindungskurve_FeCN/500uW/10/a000811.tif", path "F:/pHGradienten/2015/150416_Bindungskurve_FeCN/500uW/10/a000812.tif", path "F:/pHGradienten/2015/150416_Bindungskurve_FeCN/500uW/10/a000813.tif", path "F:/pHGradienten/2015/150416_Bindungskurve_FeCN/500uW/10/a000814.tif", path "F:/pHGradienten/2015/150416_Bindungskurve_FeCN/500uW/10/a000815.tif", path "F:/pHGradienten/2015/150416_Bindungskurve_FeCN/500uW/10/a000816.tif", path "F:/pHGradienten/2015/150416_Bindungskurve_FeCN/500uW/10/a000817.tif", path "F:/pHGradienten/2015/150416_Bindungskurve_FeCN/500uW/10/a000818.tif", path "F:/pHGradienten/2015/150416_Bindungskurve_FeCN/500uW/10/a000819.tif", path "F:/pHGradienten/2015/150416_Bindungskurve_FeCN/500uW/10/a000820.tif", path "F:/pHGradienten/2015/150416_Bindungskurve_FeCN/500uW/10/a000821.tif", path "F:/pHGradienten/2015/150416_Bindungskurve_FeCN/500uW/10/a000822.tif", path "F:/pHGradienten/2015/150416_Bindungskurve_FeCN/500uW/10/a000823.tif", path "F:/pHGradienten/2015/150416_Bindungskurve_FeCN/500uW/10/a000824.tif", path "F:/pHGradienten/2015/150416_Bindungskurve_FeCN/500uW/10/a000825.tif", path "F:/pHGradienten/2015/150416_Bindungskurve_FeCN/500uW/10/a000826.tif", path "F:/pHGradienten/2015/150416_Bindungskurve_FeCN/500uW/10/a000827.tif", path "F:/pHGradienten/2015/150416_Bindungskurve_FeCN/500uW/10/a000828.tif", path "F:/pHGradienten/2015/150416_Bindungskurve_FeCN/500uW/10/a000829.tif", path "F:/pHGradienten/2015/150416_Bindungskurve_FeCN/500uW/10/a000830.tif", path "F:/pHGradienten/2015/150416_Bindungskurve_FeCN/500uW/10/a000831.tif", path "F:/pHGradienten/2015/150416_Bindungskurve_FeCN/500uW/10/a000832.tif", path "F:/pHGradienten/2015/150416_Bindungskurve_FeCN/500uW/10/a000833.tif", path "F:/pHGradienten/2015/150416_Bindungskurve_FeCN/500uW/10/a000834.tif", path "F:/pHGradienten/2015/150416_Bindungskurve_FeCN/500uW/10/a000835.tif", path "F:/pHGradienten/2015/150416_Bindungskurve_FeCN/500uW/10/a000836.tif", path "F:/pHGradienten/2015/150416_Bindungskurve_FeCN/500uW/10/a000837.tif", path "F:/pHGradienten/2015/150416_Bindungskurve_FeCN/500uW/10/a000838.tif", path "F:/pHGradienten/2015/150416_Bindungskurve_FeCN/500uW/10/a000839.tif", path "F:/pHGradienten/2015/150416_Bindungskurve_FeCN/500uW/10/a000840.tif", path "F:/pHGradienten/2015/150416_Bindungskurve_FeCN/500uW/10/a000841.tif", path "F:/pHGradienten/2015/150416_Bindungskurve_FeCN/500uW/10/a000842.tif", path "F:/pHGradienten/2015/150416_Bindungskurve_FeCN/500uW/10/a000843.tif", path "F:/pHGradienten/2015/150416_Bindungskurve_FeCN/500uW/10/a000844.tif", path "F:/pHGradienten/2015/150416_Bindungskurve_FeCN/500uW/10/a000845.tif", path "F:/pHGradienten/2015/150416_Bindungskurve_FeCN/500uW/10/a000846.tif", path "F:/pHGradienten/2015/150416_Bindungskurve_FeCN/500uW/10/a000847.tif", path "F:/pHGradienten/2015/150416_Bindungskurve_FeCN/500uW/10/a000848.tif", path "F:/pHGradienten/2015/150416_Bindungskurve_FeCN/500uW/10/a000849.tif", path "F:/pHGradienten/2015/150416_Bindungskurve_FeCN/500uW/10/a000850.tif", path "F:/pHGradienten/2015/150416_Bindungskurve_FeCN/500uW/10/a000851.tif", path "F:/pHGradienten/2015/150416_Bindungskurve_FeCN/500uW/10/a000852.tif", path "F:/pHGradienten/2015/150416_Bindungskurve_FeCN/500uW/10/a000853.tif", path "F:/pHGradienten/2015/150416_Bindungskurve_FeCN/500uW/10/a000854.tif", path "F:/pHGradienten/2015/150416_Bindungskurve_FeCN/500uW/10/a000855.tif", path "F:/pHGradienten/2015/150416_Bindungskurve_FeCN/500uW/10/a000856.tif", path "F:/pHGradienten/2015/150416_Bindungskurve_FeCN/500uW/10/a000857.tif", path "F:/pHGradienten/2015/150416_Bindungskurve_FeCN/500uW/10/a000858.tif", path "F:/pHGradienten/2015/150416_Bindungskurve_FeCN/500uW/10/a000859.tif", path "F:/pHGradienten/2015/150416_Bindungskurve_FeCN/500uW/10/a000860.tif", path "F:/pHGradienten/2015/150416_Bindungskurve_FeCN/500uW/10/a000861.tif", path "F:/pHGradienten/2015/150416_Bindungskurve_FeCN/500uW/10/a000862.tif", path "F:/pHGradienten/2015/150416_Bindungskurve_FeCN/500uW/10/a000863.tif", path "F:/pHGradienten/2015/150416_Bindungskurve_FeCN/500uW/10/a000864.tif", path "F:/pHGradienten/2015/150416_Bindungskurve_FeCN/500uW/10/a000865.tif", path "F:/pHGradienten/2015/150416_Bindungskurve_FeCN/500uW/10/a000866.tif", path "F:/pHGradienten/2015/150416_Bindungskurve_FeCN/500uW/10/a000867.tif", path "F:/pHGradienten/2015/150416_Bindungskurve_FeCN/500uW/10/a000868.tif", path "F:/pHGradienten/2015/150416_Bindungskurve_FeCN/500uW/10/a000869.tif", path "F:/pHGradienten/2015/150416_Bindungskurve_FeCN/500uW/10/a000870.tif", path "F:/pHGradienten/2015/150416_Bindungskurve_FeCN/500uW/10/a000871.tif", path "F:/pHGradienten/2015/150416_Bindungskurve_FeCN/500uW/10/a000872.tif", path "F:/pHGradienten/2015/150416_Bindungskurve_FeCN/500uW/10/a000873.tif", path "F:/pHGradienten/2015/150416_Bindungskurve_FeCN/500uW/10/a000874.tif", path "F:/pHGradienten/2015/150416_Bindungskurve_FeCN/500uW/10/a000875.tif", path "F:/pHGradienten/2015/150416_Bindungskurve_FeCN/500uW/10/a000876.tif", path "F:/pHGradienten/2015/150416_Bindungskurve_FeCN/500uW/10/a000877.tif", path "F:/pHGradienten/2015/150416_Bindungskurve_FeCN/500uW/10/a000878.tif", path "F:/pHGradienten/2015/150416_Bindungskurve_FeCN/500uW/10/a000879.tif", path "F:/pHGradienten/2015/150416_Bindungskurve_FeCN/500uW/10/a000880.tif", path "F:/pHGradienten/2015/150416_Bindungskurve_FeCN/500uW/10/a000881.tif", path "F:/pHGradienten/2015/150416_Bindungskurve_FeCN/500uW/10/a000882.tif", path "F:/pHGradienten/2015/150416_Bindungskurve_FeCN/500uW/10/a000883.tif", path "F:/pHGradienten/2015/150416_Bindungskurve_FeCN/500uW/10/a000884.tif", path "F:/pHGradienten/2015/150416_Bindungskurve_FeCN/500uW/10/a000885.tif", path "F:/pHGradienten/2015/150416_Bindungskurve_FeCN/500uW/10/a000886.tif", path "F:/pHGradienten/2015/150416_Bindungskurve_FeCN/500uW/10/a000887.tif", path "F:/pHGradienten/2015/150416_Bindungskurve_FeCN/500uW/10/a000888.tif", path "F:/pHGradienten/2015/150416_Bindungskurve_FeCN/500uW/10/a000889.tif", path "F:/pHGradienten/2015/150416_Bindungskurve_FeCN/500uW/10/a000890.tif", path "F:/pHGradienten/2015/150416_Bindungskurve_FeCN/500uW/10/a000891.tif", path "F:/pHGradienten/2015/150416_Bindungskurve_FeCN/500uW/10/a000892.tif", path "F:/pHGradienten/2015/150416_Bindungskurve_FeCN/500uW/10/a000893.tif", path "F:/pHGradienten/2015/150416_Bindungskurve_FeCN/500uW/10/a000894.tif", path "F:/pHGradienten/2015/150416_Bindungskurve_FeCN/500uW/10/a000895.tif", path "F:/pHGradienten/2015/150416_Bindungskurve_FeCN/500uW/10/a000896.tif", path "F:/pHGradienten/2015/150416_Bindungskurve_FeCN/500uW/10/a000897.tif", path "F:/pHGradienten/2015/150416_Bindungskurve_FeCN/500uW/10/a000898.tif", path "F:/pHGradienten/2015/150416_Bindungskurve_FeCN/500uW/10/a000899.tif", path "F:/pHGradienten/2015/150416_Bindungskurve_FeCN/500uW/10/a000900.tif", path "F:/pHGradienten/2015/150416_Bindungskurve_FeCN/500uW/10/a000901.tif", path "F:/pHGradienten/2015/150416_Bindungskurve_FeCN/500uW/10/a000902.tif", path "F:/pHGradienten/2015/150416_Bindungskurve_FeCN/500uW/10/a000903.tif", path "F:/pHGradienten/2015/150416_Bindungskurve_FeCN/500uW/10/a000904.tif", path "F:/pHGradienten/2015/150416_Bindungskurve_FeCN/500uW/10/a000905.tif", path "F:/pHGradienten/2015/150416_Bindungskurve_FeCN/500uW/10/a000906.tif", path "F:/pHGradienten/2015/150416_Bindungskurve_FeCN/500uW/10/a000907.tif", path "F:/pHGradienten/2015/150416_Bindungskurve_FeCN/500uW/10/a000908.tif", path "F:/pHGradienten/2015/150416_Bindungskurve_FeCN/500uW/10/a000909.tif", path "F:/pHGradienten/2015/150416_Bindungskurve_FeCN/500uW/10/a000910.tif", path "F:/pHGradienten/2015/150416_Bindungskurve_FeCN/500uW/10/a000911.tif", path "F:/pHGradienten/2015/150416_Bindungskurve_FeCN/500uW/10/a000912.tif", path "F:/pHGradienten/2015/150416_Bindungskurve_FeCN/500uW/10/a000913.tif", path "F:/pHGradienten/2015/150416_Bindungskurve_FeCN/500uW/10/a000914.tif", path "F:/pHGradienten/2015/150416_Bindungskurve_FeCN/500uW/10/a000915.tif", path "F:/pHGradienten/2015/150416_Bindungskurve_FeCN/500uW/10/a000916.tif", path "F:/pHGradienten/2015/150416_Bindungskurve_FeCN/500uW/10/a000917.tif", path "F:/pHGradienten/2015/150416_Bindungskurve_FeCN/500uW/10/a000918.tif", path "F:/pHGradienten/2015/150416_Bindungskurve_FeCN/500uW/10/a000919.tif", path "F:/pHGradienten/2015/150416_Bindungskurve_FeCN/500uW/10/a000920.tif", path "F:/pHGradienten/2015/150416_Bindungskurve_FeCN/500uW/10/a000921.tif", path "F:/pHGradienten/2015/150416_Bindungskurve_FeCN/500uW/10/a000922.tif", path "F:/pHGradienten/2015/150416_Bindungskurve_FeCN/500uW/10/a000923.tif", path "F:/pHGradienten/2015/150416_Bindungskurve_FeCN/500uW/10/a000924.tif", path "F:/pHGradienten/2015/150416_Bindungskurve_FeCN/500uW/10/a000925.tif", path "F:/pHGradienten/2015/150416_Bindungskurve_FeCN/500uW/10/a000926.tif", path "F:/pHGradienten/2015/150416_Bindungskurve_FeCN/500uW/10/a000927.tif", path "F:/pHGradienten/2015/150416_Bindungskurve_FeCN/500uW/10/a000928.tif", path "F:/pHGradienten/2015/150416_Bindungskurve_FeCN/500uW/10/a000929.tif", path "F:/pHGradienten/2015/150416_Bindungskurve_FeCN/500uW/10/a000930.tif", path "F:/pHGradienten/2015/150416_Bindungskurve_FeCN/500uW/10/a000931.tif", path "F:/pHGradienten/2015/150416_Bindungskurve_FeCN/500uW/10/a000932.tif", path "F:/pHGradienten/2015/150416_Bindungskurve_FeCN/500uW/10/a000933.tif", path "F:/pHGradienten/2015/150416_Bindungskurve_FeCN/500uW/10/a000934.tif", path "F:/pHGradienten/2015/150416_Bindungskurve_FeCN/500uW/10/a000935.tif", path "F:/pHGradienten/2015/150416_Bindungskurve_FeCN/500uW/10/a000936.tif", path "F:/pHGradienten/2015/150416_Bindungskurve_FeCN/500uW/10/a000937.tif", path "F:/pHGradienten/2015/150416_Bindungskurve_FeCN/500uW/10/a000938.tif", path "F:/pHGradienten/2015/150416_Bindungskurve_FeCN/500uW/10/a000939.tif", path "F:/pHGradienten/2015/150416_Bindungskurve_FeCN/500uW/10/a000940.tif", path "F:/pHGradienten/2015/150416_Bindungskurve_FeCN/500uW/10/a000941.tif", path "F:/pHGradienten/2015/150416_Bindungskurve_FeCN/500uW/10/a000942.tif", path "F:/pHGradienten/2015/150416_Bindungskurve_FeCN/500uW/10/a000943.tif", path "F:/pHGradienten/2015/150416_Bindungskurve_FeCN/500uW/10/a000944.tif", path "F:/pHGradienten/2015/150416_Bindungskurve_FeCN/500uW/10/a000945.tif", path "F:/pHGradienten/2015/150416_Bindungskurve_FeCN/500uW/10/a000946.tif", path "F:/pHGradienten/2015/150416_Bindungskurve_FeCN/500uW/10/a000947.tif", path "F:/pHGradienten/2015/150416_Bindungskurve_FeCN/500uW/10/a000948.tif", path "F:/pHGradienten/2015/150416_Bindungskurve_FeCN/500uW/10/a000949.tif", path "F:/pHGradienten/2015/150416_Bindungskurve_FeCN/500uW/10/a000950.tif", path "F:/pHGradienten/2015/150416_Bindungskurve_FeCN/500uW/10/a000951.tif", path "F:/pHGradienten/2015/150416_Bindungskurve_FeCN/500uW/10/a000952.tif", path "F:/pHGradienten/2015/150416_Bindungskurve_FeCN/500uW/10/a000953.tif", path "F:/pHGradienten/2015/150416_Bindungskurve_FeCN/500uW/10/a000954.tif", path "F:/pHGradienten/2015/150416_Bindungskurve_FeCN/500uW/10/a000955.tif", path "F:/pHGradienten/2015/150416_Bindungskurve_FeCN/500uW/10/a000956.tif", path "F:/pHGradienten/2015/150416_Bindungskurve_FeCN/500uW/10/a000957.tif", path "F:/pHGradienten/2015/150416_Bindungskurve_FeCN/500uW/10/a000958.tif", path "F:/pHGradienten/2015/150416_Bindungskurve_FeCN/500uW/10/a000959.tif", path "F:/pHGradienten/2015/150416_Bindungskurve_FeCN/500uW/10/a000960.tif", path "F:/pHGradienten/2015/150416_Bindungskurve_FeCN/500uW/10/a000961.tif", path "F:/pHGradienten/2015/150416_Bindungskurve_FeCN/500uW/10/a000962.tif", path "F:/pHGradienten/2015/150416_Bindungskurve_FeCN/500uW/10/a000963.tif", path "F:/pHGradienten/2015/150416_Bindungskurve_FeCN/500uW/10/a000964.tif", path "F:/pHGradienten/2015/150416_Bindungskurve_FeCN/500uW/10/a000965.tif", path "F:/pHGradienten/2015/150416_Bindungskurve_FeCN/500uW/10/a000966.tif", path "F:/pHGradienten/2015/150416_Bindungskurve_FeCN/500uW/10/a000967.tif", path "F:/pHGradienten/2015/150416_Bindungskurve_FeCN/500uW/10/a000968.tif", path "F:/pHGradienten/2015/150416_Bindungskurve_FeCN/500uW/10/a000969.tif", path "F:/pHGradienten/2015/150416_Bindungskurve_FeCN/500uW/10/a000970.tif", path "F:/pHGradienten/2015/150416_Bindungskurve_FeCN/500uW/10/a000971.tif", path "F:/pHGradienten/2015/150416_Bindungskurve_FeCN/500uW/10/a000972.tif", path "F:/pHGradienten/2015/150416_Bindungskurve_FeCN/500uW/10/a000973.tif", path "F:/pHGradienten/2015/150416_Bindungskurve_FeCN/500uW/10/a000974.tif", path "F:/pHGradienten/2015/150416_Bindungskurve_FeCN/500uW/10/a000975.tif", path "F:/pHGradienten/2015/150416_Bindungskurve_FeCN/500uW/10/a000976.tif", path "F:/pHGradienten/2015/150416_Bindungskurve_FeCN/500uW/10/a000977.tif", path "F:/pHGradienten/2015/150416_Bindungskurve_FeCN/500uW/10/a000978.tif", path "F:/pHGradienten/2015/150416_Bindungskurve_FeCN/500uW/10/a000979.tif", path "F:/pHGradienten/2015/150416_Bindungskurve_FeCN/500uW/10/a000980.tif", path "F:/pHGradienten/2015/150416_Bindungskurve_FeCN/500uW/10/a000981.tif", path "F:/pHGradienten/2015/150416_Bindungskurve_FeCN/500uW/10/a000982.tif", path "F:/pHGradienten/2015/150416_Bindungskurve_FeCN/500uW/10/a000983.tif", path "F:/pHGradienten/2015/150416_Bindungskurve_FeCN/500uW/10/a000984.tif", path "F:/pHGradienten/2015/150416_Bindungskurve_FeCN/500uW/10/a000985.tif", path "F:/pHGradienten/2015/150416_Bindungskurve_FeCN/500uW/10/a000986.tif", path "F:/pHGradienten/2015/150416_Bindungskurve_FeCN/500uW/10/a000987.tif", path "F:/pHGradienten/2015/150416_Bindungskurve_FeCN/500uW/10/a000988.tif", path "F:/pHGradienten/2015/150416_Bindungskurve_FeCN/500uW/10/a000989.tif", path "F:/pHGradienten/2015/150416_Bindungskurve_FeCN/500uW/10/a000990.tif", path "F:/pHGradienten/2015/150416_Bindungskurve_FeCN/500uW/10/a000991.tif", path "F:/pHGradienten/2015/150416_Bindungskurve_FeCN/500uW/10/a000992.tif", path "F:/pHGradienten/2015/150416_Bindungskurve_FeCN/500uW/10/a000993.tif", path "F:/pHGradienten/2015/150416_Bindungskurve_FeCN/500uW/10/a000994.tif", path "F:/pHGradienten/2015/150416_Bindungskurve_FeCN/500uW/10/a000995.tif", path "F:/pHGradienten/2015/150416_Bindungskurve_FeCN/500uW/10/a000996.tif", path "F:/pHGradienten/2015/150416_Bindungskurve_FeCN/500uW/10/a000997.tif", path "F:/pHGradienten/2015/150416_Bindungskurve_FeCN/500uW/10/a000998.tif", path "F:/pHGradienten/2015/150416_Bindungskurve_FeCN/500uW/10/a000999.tif", path "F:/pHGradienten/2015/150416_Bindungskurve_FeCN/500uW/10/a001000.tif", path "F:/pHGradienten/2015/150416_Bindungskurve_FeCN/500uW/10/a001001.tif", path "F:/pHGradienten/2015/150416_Bindungskurve_FeCN/500uW/10/a001002.tif", path "F:/pHGradienten/2015/150416_Bindungskurve_FeCN/500uW/10/a001003.tif", path "F:/pHGradienten/2015/150416_Bindungskurve_FeCN/500uW/10/a001004.tif", path "F:/pHGradienten/2015/150416_Bindungskurve_FeCN/500uW/10/a001005.tif", path "F:/pHGradienten/2015/150416_Bindungskurve_FeCN/500uW/10/a001006.tif", path "F:/pHGradienten/2015/150416_Bindungskurve_FeCN/500uW/10/a001007.tif", path "F:/pHGradienten/2015/150416_Bindungskurve_FeCN/500uW/10/a001008.tif", path "F:/pHGradienten/2015/150416_Bindungskurve_FeCN/500uW/10/a001009.tif", path "F:/pHGradienten/2015/150416_Bindungskurve_FeCN/500uW/10/a001010.tif", path "F:/pHGradienten/2015/150416_Bindungskurve_FeCN/500uW/10/a001011.tif", path "F:/pHGradienten/2015/150416_Bindungskurve_FeCN/500uW/10/a001012.tif", path "F:/pHGradienten/2015/150416_Bindungskurve_FeCN/500uW/10/a001013.tif", path "F:/pHGradienten/2015/150416_Bindungskurve_FeCN/500uW/10/a001014.tif", path "F:/pHGradienten/2015/150416_Bindungskurve_FeCN/500uW/10/a001015.tif", path "F:/pHGradienten/2015/150416_Bindungskurve_FeCN/500uW/10/a001016.tif", path "F:/pHGradienten/2015/150416_Bindungskurve_FeCN/500uW/10/a001017.tif", path "F:/pHGradienten/2015/150416_Bindungskurve_FeCN/500uW/10/a001018.tif", path "F:/pHGradienten/2015/150416_Bindungskurve_FeCN/500uW/10/a001019.tif", path "F:/pHGradienten/2015/150416_Bindungskurve_FeCN/500uW/10/a001020.tif", path "F:/pHGradienten/2015/150416_Bindungskurve_FeCN/500uW/10/a001021.tif", path "F:/pHGradienten/2015/150416_Bindungskurve_FeCN/500uW/10/a001022.tif", path "F:/pHGradienten/2015/150416_Bindungskurve_FeCN/500uW/10/a001023.tif", path "F:/pHGradienten/2015/150416_Bindungskurve_FeCN/500uW/10/a001024.tif", path "F:/pHGradienten/2015/150416_Bindungskurve_FeCN/500uW/10/a001025.tif", path "F:/pHGradienten/2015/150416_Bindungskurve_FeCN/500uW/10/a001026.tif", path "F:/pHGradienten/2015/150416_Bindungskurve_FeCN/500uW/10/a001027.tif", path "F:/pHGradienten/2015/150416_Bindungskurve_FeCN/500uW/10/a001028.tif", path "F:/pHGradienten/2015/150416_Bindungskurve_FeCN/500uW/10/a001029.tif", path "F:/pHGradienten/2015/150416_Bindungskurve_FeCN/500uW/10/a001030.tif", path "F:/pHGradienten/2015/150416_Bindungskurve_FeCN/500uW/10/a001031.tif", path "F:/pHGradienten/2015/150416_Bindungskurve_FeCN/500uW/10/a001032.tif", path "F:/pHGradienten/2015/150416_Bindungskurve_FeCN/500uW/10/a001033.tif", path "F:/pHGradienten/2015/150416_Bindungskurve_FeCN/500uW/10/a001034.tif", path "F:/pHGradienten/2015/150416_Bindungskurve_FeCN/500uW/10/a001035.tif", path "F:/pHGradienten/2015/150416_Bindungskurve_FeCN/500uW/10/a001036.tif", path "F:/pHGradienten/2015/150416_Bindungskurve_FeCN/500uW/10/a001037.tif", path "F:/pHGradienten/2015/150416_Bindungskurve_FeCN/500uW/10/a001038.tif", path "F:/pHGradienten/2015/150416_Bindungskurve_FeCN/500uW/10/a001039.tif", path "F:/pHGradienten/2015/150416_Bindungskurve_FeCN/500uW/10/a001040.tif", path "F:/pHGradienten/2015/150416_Bindungskurve_FeCN/500uW/10/a001041.tif", path "F:/pHGradienten/2015/150416_Bindungskurve_FeCN/500uW/10/a001042.tif", path "F:/pHGradienten/2015/150416_Bindungskurve_FeCN/500uW/10/a001043.tif", path "F:/pHGradienten/2015/150416_Bindungskurve_FeCN/500uW/10/a001044.tif", path "F:/pHGradienten/2015/150416_Bindungskurve_FeCN/500uW/10/a001045.tif", path "F:/pHGradienten/2015/150416_Bindungskurve_FeCN/500uW/10/a001046.tif", path "F:/pHGradienten/2015/150416_Bindungskurve_FeCN/500uW/10/a001047.tif", path "F:/pHGradienten/2015/150416_Bindungskurve_FeCN/500uW/10/a001048.tif", path "F:/pHGradienten/2015/150416_Bindungskurve_FeCN/500uW/10/a001049.tif", path "F:/pHGradienten/2015/150416_Bindungskurve_FeCN/500uW/10/a001050.tif", path "F:/pHGradienten/2015/150416_Bindungskurve_FeCN/500uW/10/a001051.tif", path "F:/pHGradienten/2015/150416_Bindungskurve_FeCN/500uW/10/a001052.tif", path "F:/pHGradienten/2015/150416_Bindungskurve_FeCN/500uW/10/a001053.tif", path "F:/pHGradienten/2015/150416_Bindungskurve_FeCN/500uW/10/a001054.tif", path "F:/pHGradienten/2015/150416_Bindungskurve_FeCN/500uW/10/a001055.tif", path "F:/pHGradienten/2015/150416_Bindungskurve_FeCN/500uW/10/a001056.tif", path "F:/pHGradienten/2015/150416_Bindungskurve_FeCN/500uW/10/a001057.tif", path "F:/pHGradienten/2015/150416_Bindungskurve_FeCN/500uW/10/a001058.tif", path "F:/pHGradienten/2015/150416_Bindungskurve_FeCN/500uW/10/a001059.tif", path "F:/pHGradienten/2015/150416_Bindungskurve_FeCN/500uW/10/a001060.tif", path "F:/pHGradienten/2015/150416_Bindungskurve_FeCN/500uW/10/a001061.tif", path "F:/pHGradienten/2015/150416_Bindungskurve_FeCN/500uW/10/a001062.tif", path "F:/pHGradienten/2015/150416_Bindungskurve_FeCN/500uW/10/a001063.tif", path "F:/pHGradienten/2015/150416_Bindungskurve_FeCN/500uW/10/a001064.tif", path "F:/pHGradienten/2015/150416_Bindungskurve_FeCN/500uW/10/a001065.tif", path "F:/pHGradienten/2015/150416_Bindungskurve_FeCN/500uW/10/a001066.tif", path "F:/pHGradienten/2015/150416_Bindungskurve_FeCN/500uW/10/a001067.tif", path "F:/pHGradienten/2015/150416_Bindungskurve_FeCN/500uW/10/a001068.tif", path "F:/pHGradienten/2015/150416_Bindungskurve_FeCN/500uW/10/a001069.tif", path "F:/pHGradienten/2015/150416_Bindungskurve_FeCN/500uW/10/a001070.tif", path "F:/pHGradienten/2015/150416_Bindungskurve_FeCN/500uW/10/a001071.tif", path "F:/pHGradienten/2015/150416_Bindungskurve_FeCN/500uW/10/a001072.tif", path "F:/pHGradienten/2015/150416_Bindungskurve_FeCN/500uW/10/a001073.tif", path "F:/pHGradienten/2015/150416_Bindungskurve_FeCN/500uW/10/a001074.tif", path "F:/pHGradienten/2015/150416_Bindungskurve_FeCN/500uW/10/a001075.tif", path "F:/pHGradienten/2015/150416_Bindungskurve_FeCN/500uW/10/a001076.tif", path "F:/pHGradienten/2015/150416_Bindungskurve_FeCN/500uW/10/a001077.tif", path "F:/pHGradienten/2015/150416_Bindungskurve_FeCN/500uW/10/a001078.tif", path "F:/pHGradienten/2015/150416_Bindungskurve_FeCN/500uW/10/a001079.tif", path "F:/pHGradienten/2015/150416_Bindungskurve_FeCN/500uW/10/a001080.tif", path "F:/pHGradienten/2015/150416_Bindungskurve_FeCN/500uW/10/a001081.tif", path "F:/pHGradienten/2015/150416_Bindungskurve_FeCN/500uW/10/a001082.tif", path "F:/pHGradienten/2015/150416_Bindungskurve_FeCN/500uW/10/a001083.tif", path "F:/pHGradienten/2015/150416_Bindungskurve_FeCN/500uW/10/a001084.tif", path "F:/pHGradienten/2015/150416_Bindungskurve_FeCN/500uW/10/a001085.tif", path "F:/pHGradienten/2015/150416_Bindungskurve_FeCN/500uW/10/a001086.tif", path "F:/pHGradienten/2015/150416_Bindungskurve_FeCN/500uW/10/a001087.tif", path "F:/pHGradienten/2015/150416_Bindungskurve_FeCN/500uW/10/a001088.tif", path "F:/pHGradienten/2015/150416_Bindungskurve_FeCN/500uW/10/a001089.tif", path "F:/pHGradienten/2015/150416_Bindungskurve_FeCN/500uW/10/a001090.tif", path "F:/pHGradienten/2015/150416_Bindungskurve_FeCN/500uW/10/a001091.tif", path "F:/pHGradienten/2015/150416_Bindungskurve_FeCN/500uW/10/a001092.tif", path "F:/pHGradienten/2015/150416_Bindungskurve_FeCN/500uW/10/a001093.tif", path "F:/pHGradienten/2015/150416_Bindungskurve_FeCN/500uW/10/a001094.tif", path "F:/pHGradienten/2015/150416_Bindungskurve_FeCN/500uW/10/a001095.tif", path "F:/pHGradienten/2015/150416_Bindungskurve_FeCN/500uW/10/a001096.tif", path "F:/pHGradienten/2015/150416_Bindungskurve_FeCN/500uW/10/a001097.tif", path "F:/pHGradienten/2015/150416_Bindungskurve_FeCN/500uW/10/a001098.tif", path "F:/pHGradienten/2015/150416_Bindungskurve_FeCN/500uW/10/a001099.tif", path "F:/pHGradienten/2015/150416_Bindungskurve_FeCN/500uW/10/a001100.tif", path "F:/pHGradienten/2015/150416_Bindungskurve_FeCN/500uW/10/a001101.tif", path "F:/pHGradienten/2015/150416_Bindungskurve_FeCN/500uW/10/a001102.tif", path "F:/pHGradienten/2015/150416_Bindungskurve_FeCN/500uW/10/a001103.tif", path "F:/pHGradienten/2015/150416_Bindungskurve_FeCN/500uW/10/a001104.tif", path "F:/pHGradienten/2015/150416_Bindungskurve_FeCN/500uW/10/a001105.tif", path "F:/pHGradienten/2015/150416_Bindungskurve_FeCN/500uW/10/a001106.tif", path "F:/pHGradienten/2015/150416_Bindungskurve_FeCN/500uW/10/a001107.tif", path "F:/pHGradienten/2015/150416_Bindungskurve_FeCN/500uW/10/a001108.tif", path "F:/pHGradienten/2015/150416_Bindungskurve_FeCN/500uW/10/a001109.tif", path "F:/pHGradienten/2015/150416_Bindungskurve_FeCN/500uW/10/a001110.tif", path "F:/pHGradienten/2015/150416_Bindungskurve_FeCN/500uW/10/a001111.tif", path "F:/pHGradienten/2015/150416_Bindungskurve_FeCN/500uW/10/a001112.tif", path "F:/pHGradienten/2015/150416_Bindungskurve_FeCN/500uW/10/a001113.tif", path "F:/pHGradienten/2015/150416_Bindungskurve_FeCN/500uW/10/a001114.tif", path "F:/pHGradienten/2015/150416_Bindungskurve_FeCN/500uW/10/a001115.tif", path "F:/pHGradienten/2015/150416_Bindungskurve_FeCN/500uW/10/a001116.tif", path "F:/pHGradienten/2015/150416_Bindungskurve_FeCN/500uW/10/a001117.tif", path "F:/pHGradienten/2015/150416_Bindungskurve_FeCN/500uW/10/a001118.tif", path "F:/pHGradienten/2015/150416_Bindungskurve_FeCN/500uW/10/a001119.tif", path "F:/pHGradienten/2015/150416_Bindungskurve_FeCN/500uW/10/a001120.tif", path "F:/pHGradienten/2015/150416_Bindungskurve_FeCN/500uW/10/a001121.tif", path "F:/pHGradienten/2015/150416_Bindungskurve_FeCN/500uW/10/a001122.tif", path "F:/pHGradienten/2015/150416_Bindungskurve_FeCN/500uW/10/a001123.tif", path "F:/pHGradienten/2015/150416_Bindungskurve_FeCN/500uW/10/a001124.tif", path "F:/pHGradienten/2015/150416_Bindungskurve_FeCN/500uW/10/a001125.tif", path "F:/pHGradienten/2015/150416_Bindungskurve_FeCN/500uW/10/a001126.tif", path "F:/pHGradienten/2015/150416_Bindungskurve_FeCN/500uW/10/a001127.tif", path "F:/pHGradienten/2015/150416_Bindungskurve_FeCN/500uW/10/a001128.tif", path "F:/pHGradienten/2015/150416_Bindungskurve_FeCN/500uW/10/a001129.tif", path "F:/pHGradienten/2015/150416_Bindungskurve_FeCN/500uW/10/a001130.tif", path "F:/pHGradienten/2015/150416_Bindungskurve_FeCN/500uW/10/a001131.tif", path "F:/pHGradienten/2015/150416_Bindungskurve_FeCN/500uW/10/a001132.tif", path "F:/pHGradienten/2015/150416_Bindungskurve_FeCN/500uW/10/a001133.tif", path "F:/pHGradienten/2015/150416_Bindungskurve_FeCN/500uW/10/a001134.tif", path "F:/pHGradienten/2015/150416_Bindungskurve_FeCN/500uW/10/a001135.tif", path "F:/pHGradienten/2015/150416_Bindungskurve_FeCN/500uW/10/a001136.tif", path "F:/pHGradienten/2015/150416_Bindungskurve_FeCN/500uW/10/a001137.tif", path "F:/pHGradienten/2015/150416_Bindungskurve_FeCN/500uW/10/a001138.tif", path "F:/pHGradienten/2015/150416_Bindungskurve_FeCN/500uW/10/a001139.tif", path "F:/pHGradienten/2015/150416_Bindungskurve_FeCN/500uW/10/a001140.tif", path "F:/pHGradienten/2015/150416_Bindungskurve_FeCN/500uW/10/a001141.tif", path "F:/pHGradienten/2015/150416_Bindungskurve_FeCN/500uW/10/a001142.tif", path "F:/pHGradienten/2015/150416_Bindungskurve_FeCN/500uW/10/a001143.tif", path "F:/pHGradienten/2015/150416_Bindungskurve_FeCN/500uW/10/a001144.tif", path "F:/pHGradienten/2015/150416_Bindungskurve_FeCN/500uW/10/a001145.tif", path "F:/pHGradienten/2015/150416_Bindungskurve_FeCN/500uW/10/a001146.tif", path "F:/pHGradienten/2015/150416_Bindungskurve_FeCN/500uW/10/a001147.tif", path "F:/pHGradienten/2015/150416_Bindungskurve_FeCN/500uW/10/a001148.tif", path "F:/pHGradienten/2015/150416_Bindungskurve_FeCN/500uW/10/a001149.tif", path "F:/pHGradienten/2015/150416_Bindungskurve_FeCN/500uW/10/a001150.tif", path "F:/pHGradienten/2015/150416_Bindungskurve_FeCN/500uW/10/a001151.tif", path "F:/pHGradienten/2015/150416_Bindungskurve_FeCN/500uW/10/a001152.tif", path "F:/pHGradienten/2015/150416_Bindungskurve_FeCN/500uW/10/a001153.tif", path "F:/pHGradienten/2015/150416_Bindungskurve_FeCN/500uW/10/a001154.tif", path "F:/pHGradienten/2015/150416_Bindungskurve_FeCN/500uW/10/a001155.tif", path "F:/pHGradienten/2015/150416_Bindungskurve_FeCN/500uW/10/a001156.tif", path "F:/pHGradienten/2015/150416_Bindungskurve_FeCN/500uW/10/a001157.tif", path "F:/pHGradienten/2015/150416_Bindungskurve_FeCN/500uW/10/a001158.tif", path "F:/pHGradienten/2015/150416_Bindungskurve_FeCN/500uW/10/a001159.tif", path "F:/pHGradienten/2015/150416_Bindungskurve_FeCN/500uW/10/a001160.tif", path "F:/pHGradienten/2015/150416_Bindungskurve_FeCN/500uW/10/a001161.tif", path "F:/pHGradienten/2015/150416_Bindungskurve_FeCN/500uW/10/a001162.tif", path "F:/pHGradienten/2015/150416_Bindungskurve_FeCN/500uW/10/a001163.tif", path "F:/pHGradienten/2015/150416_Bindungskurve_FeCN/500uW/10/a001164.tif", path "F:/pHGradienten/2015/150416_Bindungskurve_FeCN/500uW/10/a001165.tif", path "F:/pHGradienten/2015/150416_Bindungskurve_FeCN/500uW/10/a001166.tif", path "F:/pHGradienten/2015/150416_Bindungskurve_FeCN/500uW/10/a001167.tif", path "F:/pHGradienten/2015/150416_Bindungskurve_FeCN/500uW/10/a001168.tif", path "F:/pHGradienten/2015/150416_Bindungskurve_FeCN/500uW/10/a001169.tif", path "F:/pHGradienten/2015/150416_Bindungskurve_FeCN/500uW/10/a001170.tif", path "F:/pHGradienten/2015/150416_Bindungskurve_FeCN/500uW/10/a001171.tif", path "F:/pHGradienten/2015/150416_Bindungskurve_FeCN/500uW/10/a001172.tif", path "F:/pHGradienten/2015/150416_Bindungskurve_FeCN/500uW/10/a001173.tif", path "F:/pHGradienten/2015/150416_Bindungskurve_FeCN/500uW/10/a001174.tif", path "F:/pHGradienten/2015/150416_Bindungskurve_FeCN/500uW/10/a001175.tif", path "F:/pHGradienten/2015/150416_Bindungskurve_FeCN/500uW/10/a001176.tif", path "F:/pHGradienten/2015/150416_Bindungskurve_FeCN/500uW/10/a001177.tif", path "F:/pHGradienten/2015/150416_Bindungskurve_FeCN/500uW/10/a001178.tif", path "F:/pHGradienten/2015/150416_Bindungskurve_FeCN/500uW/10/a001179.tif", path "F:/pHGradienten/2015/150416_Bindungskurve_FeCN/500uW/10/a001180.tif", path "F:/pHGradienten/2015/150416_Bindungskurve_FeCN/500uW/10/a001181.tif", path "F:/pHGradienten/2015/150416_Bindungskurve_FeCN/500uW/10/a001182.tif", path "F:/pHGradienten/2015/150416_Bindungskurve_FeCN/500uW/10/a001183.tif", path "F:/pHGradienten/2015/150416_Bindungskurve_FeCN/500uW/10/a001184.tif", path "F:/pHGradienten/2015/150416_Bindungskurve_FeCN/500uW/10/a001185.tif", path "F:/pHGradienten/2015/150416_Bindungskurve_FeCN/500uW/10/a001186.tif", path "F:/pHGradienten/2015/150416_Bindungskurve_FeCN/500uW/10/a001187.tif", path "F:/pHGradienten/2015/150416_Bindungskurve_FeCN/500uW/10/a001188.tif", path "F:/pHGradienten/2015/150416_Bindungskurve_FeCN/500uW/10/a001189.tif", path "F:/pHGradienten/2015/150416_Bindungskurve_FeCN/500uW/10/a001190.tif", path "F:/pHGradienten/2015/150416_Bindungskurve_FeCN/500uW/10/a001191.tif", path "F:/pHGradienten/2015/150416_Bindungskurve_FeCN/500uW/10/a001192.tif", path "F:/pHGradienten/2015/150416_Bindungskurve_FeCN/500uW/10/a001193.tif", path "F:/pHGradienten/2015/150416_Bindungskurve_FeCN/500uW/10/a001194.tif", path "F:/pHGradienten/2015/150416_Bindungskurve_FeCN/500uW/10/a001195.tif", path "F:/pHGradienten/2015/150416_Bindungskurve_FeCN/500uW/10/a001196.tif", path "F:/pHGradienten/2015/150416_Bindungskurve_FeCN/500uW/10/a001197.tif", path "F:/pHGradienten/2015/150416_Bindungskurve_FeCN/500uW/10/a001198.tif", path "F:/pHGradienten/2015/150416_Bindungskurve_FeCN/500uW/10/a001199.tif", path "F:/pHGradienten/2015/150416_Bindungskurve_FeCN/500uW/10/a001200.tif", path "F:/pHGradienten/2015/150416_Bindungskurve_FeCN/500uW/10/a001201.tif", path "F:/pHGradienten/2015/150416_Bindungskurve_FeCN/500uW/10/a001202.tif", path "F:/pHGradienten/2015/150416_Bindungskurve_FeCN/500uW/10/a001203.tif", path "F:/pHGradienten/2015/150416_Bindungskurve_FeCN/500uW/10/a001204.tif", path "F:/pHGradienten/2015/150416_Bindungskurve_FeCN/500uW/10/a001205.tif", path "F:/pHGradienten/2015/150416_Bindungskurve_FeCN/500uW/10/a001206.tif", path "F:/pHGradienten/2015/150416_Bindungskurve_FeCN/500uW/10/a001207.tif", path "F:/pHGradienten/2015/150416_Bindungskurve_FeCN/500uW/10/a001208.tif", path "F:/pHGradienten/2015/150416_Bindungskurve_FeCN/500uW/10/a001209.tif", path "F:/pHGradienten/2015/150416_Bindungskurve_FeCN/500uW/10/a001210.tif", path "F:/pHGradienten/2015/150416_Bindungskurve_FeCN/500uW/10/a001211.tif", path "F:/pHGradienten/2015/150416_Bindungskurve_FeCN/500uW/10/a001212.tif", path "F:/pHGradienten/2015/150416_Bindungskurve_FeCN/500uW/10/a001213.tif", path "F:/pHGradienten/2015/150416_Bindungskurve_FeCN/500uW/10/a001214.tif", path "F:/pHGradienten/2015/150416_Bindungskurve_FeCN/500uW/10/a001215.tif", path "F:/pHGradienten/2015/150416_Bindungskurve_FeCN/500uW/10/a001216.tif", path "F:/pHGradienten/2015/150416_Bindungskurve_FeCN/500uW/10/a001217.tif", path "F:/pHGradienten/2015/150416_Bindungskurve_FeCN/500uW/10/a001218.tif", path "F:/pHGradienten/2015/150416_Bindungskurve_FeCN/500uW/10/a001219.tif", path "F:/pHGradienten/2015/150416_Bindungskurve_FeCN/500uW/10/a001220.tif", path "F:/pHGradienten/2015/150416_Bindungskurve_FeCN/500uW/10/a001221.tif", path "F:/pHGradienten/2015/150416_Bindungskurve_FeCN/500uW/10/a001222.tif", path "F:/pHGradienten/2015/150416_Bindungskurve_FeCN/500uW/10/a001223.tif", path "F:/pHGradienten/2015/150416_Bindungskurve_FeCN/500uW/10/a001224.tif", path "F:/pHGradienten/2015/150416_Bindungskurve_FeCN/500uW/10/a001225.tif", path "F:/pHGradienten/2015/150416_Bindungskurve_FeCN/500uW/10/a001226.tif", path "F:/pHGradienten/2015/150416_Bindungskurve_FeCN/500uW/10/a001227.tif", path "F:/pHGradienten/2015/150416_Bindungskurve_FeCN/500uW/10/a001228.tif", path "F:/pHGradienten/2015/150416_Bindungskurve_FeCN/500uW/10/a001229.tif", path "F:/pHGradienten/2015/150416_Bindungskurve_FeCN/500uW/10/a001230.tif", path "F:/pHGradienten/2015/150416_Bindungskurve_FeCN/500uW/10/a001231.tif", path "F:/pHGradienten/2015/150416_Bindungskurve_FeCN/500uW/10/a001232.tif", path "F:/pHGradienten/2015/150416_Bindungskurve_FeCN/500uW/10/a001233.tif", path "F:/pHGradienten/2015/150416_Bindungskurve_FeCN/500uW/10/a001234.tif", path "F:/pHGradienten/2015/150416_Bindungskurve_FeCN/500uW/10/a001235.tif", path "F:/pHGradienten/2015/150416_Bindungskurve_FeCN/500uW/10/a001236.tif", path "F:/pHGradienten/2015/150416_Bindungskurve_FeCN/500uW/10/a001237.tif", path "F:/pHGradienten/2015/150416_Bindungskurve_FeCN/500uW/10/a001238.tif", path "F:/pHGradienten/2015/150416_Bindungskurve_FeCN/500uW/10/a001239.tif", path "F:/pHGradienten/2015/150416_Bindungskurve_FeCN/500uW/10/a001240.tif", path "F:/pHGradienten/2015/150416_Bindungskurve_FeCN/500uW/10/a001241.tif", path "F:/pHGradienten/2015/150416_Bindungskurve_FeCN/500uW/10/a001242.tif", path "F:/pHGradienten/2015/150416_Bindungskurve_FeCN/500uW/10/a001243.tif", path "F:/pHGradienten/2015/150416_Bindungskurve_FeCN/500uW/10/a001244.tif", path "F:/pHGradienten/2015/150416_Bindungskurve_FeCN/500uW/10/a001245.tif", path "F:/pHGradienten/2015/150416_Bindungskurve_FeCN/500uW/10/a001246.tif", path "F:/pHGradienten/2015/150416_Bindungskurve_FeCN/500uW/10/a001247.tif", path "F:/pHGradienten/2015/150416_Bindungskurve_FeCN/500uW/10/a001248.tif", path "F:/pHGradienten/2015/150416_Bindungskurve_FeCN/500uW/10/a001249.tif", path "F:/pHGradienten/2015/150416_Bindungskurve_FeCN/500uW/10/a001250.tif", path "F:/pHGradienten/2015/150416_Bindungskurve_FeCN/500uW/10/a001251.tif", path "F:/pHGradienten/2015/150416_Bindungskurve_FeCN/500uW/10/a001252.tif", path "F:/pHGradienten/2015/150416_Bindungskurve_FeCN/500uW/10/a001253.tif", path "F:/pHGradienten/2015/150416_Bindungskurve_FeCN/500uW/10/a001254.tif", path "F:/pHGradienten/2015/150416_Bindungskurve_FeCN/500uW/10/a001255.tif", path "F:/pHGradienten/2015/150416_Bindungskurve_FeCN/500uW/10/a001256.tif", path "F:/pHGradienten/2015/150416_Bindungskurve_FeCN/500uW/10/a001257.tif", path "F:/pHGradienten/2015/150416_Bindungskurve_FeCN/500uW/10/a001258.tif", path "F:/pHGradienten/2015/150416_Bindungskurve_FeCN/500uW/10/a001259.tif", path "F:/pHGradienten/2015/150416_Bindungskurve_FeCN/500uW/10/a001260.tif", path "F:/pHGradienten/2015/150416_Bindungskurve_FeCN/500uW/10/a001261.tif", path "F:/pHGradienten/2015/150416_Bindungskurve_FeCN/500uW/10/a001262.tif", path "F:/pHGradienten/2015/150416_Bindungskurve_FeCN/500uW/10/a001263.tif", path "F:/pHGradienten/2015/150416_Bindungskurve_FeCN/500uW/10/a001264.tif", path "F:/pHGradienten/2015/150416_Bindungskurve_FeCN/500uW/10/a001265.tif", path "F:/pHGradienten/2015/150416_Bindungskurve_FeCN/500uW/10/a001266.tif", path "F:/pHGradienten/2015/150416_Bindungskurve_FeCN/500uW/10/a001267.tif", path "F:/pHGradienten/2015/150416_Bindungskurve_FeCN/500uW/10/a001268.tif", path "F:/pHGradienten/2015/150416_Bindungskurve_FeCN/500uW/10/a001269.tif", path "F:/pHGradienten/2015/150416_Bindungskurve_FeCN/500uW/10/a001270.tif", path "F:/pHGradienten/2015/150416_Bindungskurve_FeCN/500uW/10/a001271.tif", path "F:/pHGradienten/2015/150416_Bindungskurve_FeCN/500uW/10/a001272.tif", path "F:/pHGradienten/2015/150416_Bindungskurve_FeCN/500uW/10/a001273.tif", path "F:/pHGradienten/2015/150416_Bindungskurve_FeCN/500uW/10/a001274.tif", path "F:/pHGradienten/2015/150416_Bindungskurve_FeCN/500uW/10/a001275.tif", path "F:/pHGradienten/2015/150416_Bindungskurve_FeCN/500uW/10/a001276.tif", path "F:/pHGradienten/2015/150416_Bindungskurve_FeCN/500uW/10/a001277.tif", path "F:/pHGradienten/2015/150416_Bindungskurve_FeCN/500uW/10/a001278.tif", path "F:/pHGradienten/2015/150416_Bindungskurve_FeCN/500uW/10/a001279.tif", path "F:/pHGradienten/2015/150416_Bindungskurve_FeCN/500uW/10/a001280.tif"]
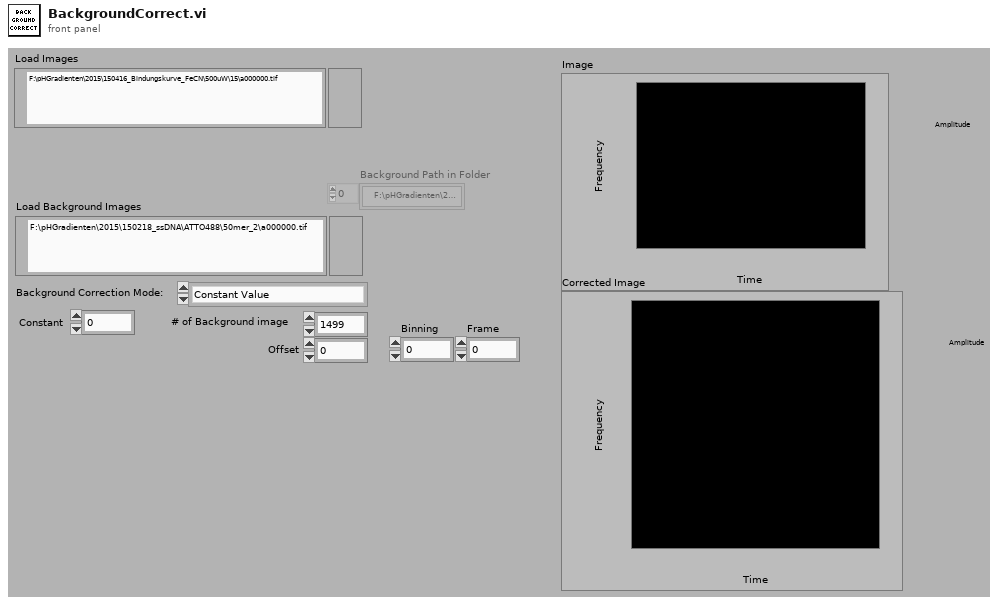
[diagram p1: front panel]
types:
  T1 = enum16{"Image by Image", "Single Image", "Single Image from Background", "Constant Value"}
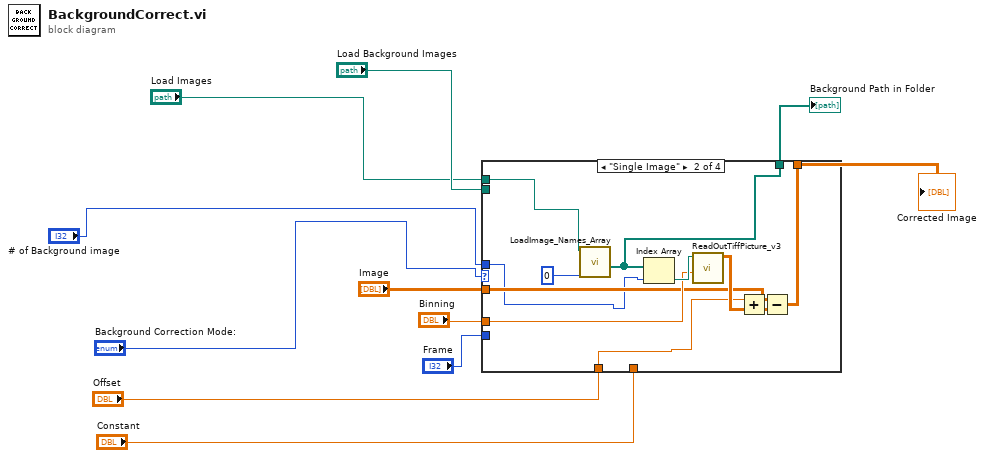
[diagram p0: block diagram]
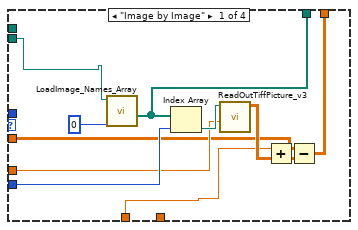
[diagram p2: hidden frame]
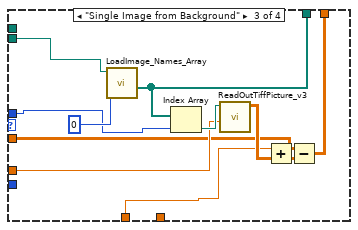
[diagram p3: hidden frame]
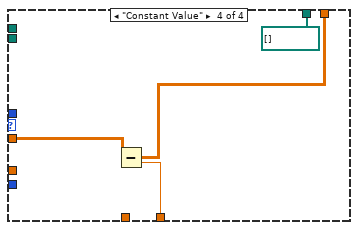
[diagram p4: hidden frame]
diagram:
  n1 = case shown="\"Single Image\"" "Background Correction Mode:" {
    tunnel: "Image" -> [w17 w29 w40 w48]
    tunnel: "Frame" -> [w20 _ _ _]
    tunnel: "Binning" -> [w19 w31 w42 _]
    tunnel: [w15 w27 w38 w47] -> w1
    tunnel: "# of Background image" -> [_ w24 w37 _]
    tunnel: "Load Background Images" -> [w14 _ w36 _]
    tunnel: [w12 w26 w35 path[] [] ("Paths")] -> w5
    tunnel: "Offset" -> [w13 w23 w34 _]
    tunnel: "Constant" -> [_ _ _ w46]
    tunnel: "Load Images" -> [_ w25 _ _]
    frame "Image by Image" {
      n2 = call "LoadImage_Names_Array.vi"("First Image"=0, "Sample Image"=w14) -> ("Paths"=w12:path[])  [unwired: 7 in, 2 out]
      n3 = Index Array(array=w12, index=w20) -> (element=w22:path)
      n4 = call "ReadOutTiffPicture_v3.vi"("Binning size"=w19, "Path"=w22) -> ("Indicator"=w18:dbl[][])  [unwired: 2 in, 3 out]
      n5 = Add(x=w13, y=w18) -> (x+y=w16:dbl[][])
      n6 = Subtract(x=w17, y=w16) -> (x-y=w15:dbl[][])
    }
    frame "Single Image" {
      n7 = call "LoadImage_Names_Array.vi"("First Image"=0, "Sample Image"=w25) -> ("Paths"=w26:path[])  [unwired: 7 in, 2 out]
      n8 = Index Array(array=w26, index=w24) -> (element=w33:path)
      n9 = call "ReadOutTiffPicture_v3.vi"("Binning size"=w31, "Path"=w33) -> ("Indicator"=w30:dbl[][])  [unwired: 2 in, 3 out]
      n10 = Add(x=w23, y=w30) -> (x+y=w28:dbl[][])
      n11 = Subtract(x=w29, y=w28) -> (x-y=w27:dbl[][])
    }
    frame "Single Image from Background" {
      n12 = call "LoadImage_Names_Array.vi"("First Image"=0, "Sample Image"=w36) -> ("Paths"=w35:path[])  [unwired: 7 in, 2 out]
      n13 = Index Array(array=w35, index=w37) -> (element=w44:path)
      n14 = call "ReadOutTiffPicture_v3.vi"("Binning size"=w42, "Path"=w44) -> ("Indicator"=w41:dbl[][])  [unwired: 2 in, 3 out]
      n15 = Add(x=w34, y=w41) -> (x+y=w39:dbl[][])
      n16 = Subtract(x=w40, y=w39) -> (x-y=w38:dbl[][])
    }
    frame "Constant Value" {
      n17 = Subtract(x=w48, y=w46) -> (x-y=w47:dbl[][])
    }
  }
  "Background Path in Folder" <- w5
  "Corrected Image" <- w1
